vi "Getdata Loop.vi"(6 "Cluster Of Graphs":T1, 8 "error in":errorcluster, 9 "Reference For PLot":T2, 10 "User Event References":T3) -> (0 "error out":errorcluster)   [LabVIEW 2015]
uses:
  TypeDef/User Event References.ctl
  TypeDef/GetData Cluster.ctl
  TypeDef/ResultUpdate Cluster.ctl
  TypeDef/Initialize_Cluster.ctl
  TypeDef/OverWrite JSON Cluster.ctl
  TypeDef/UE Reference For Plot.ctl
  TypeDef/Plot Cluster.ctl
  TypeDef/GraphReff.ctl
  <vilib>/event_ctls.llb/usereventprio.ctl
  TypeDef/Shift Registers Cluster.ctl
  TypeDef/JSON Cluster(Int).ctl
  <vilib>/Utility/file.llb/Write Delimited Spreadsheet (string).vi
panel:
  out "Default Update Rate  3":enum16{"HIGH", "MEDIUM", "LOW"}(ring)
  out "Get Data Active 2":bool
  # "GetData Test Bench"
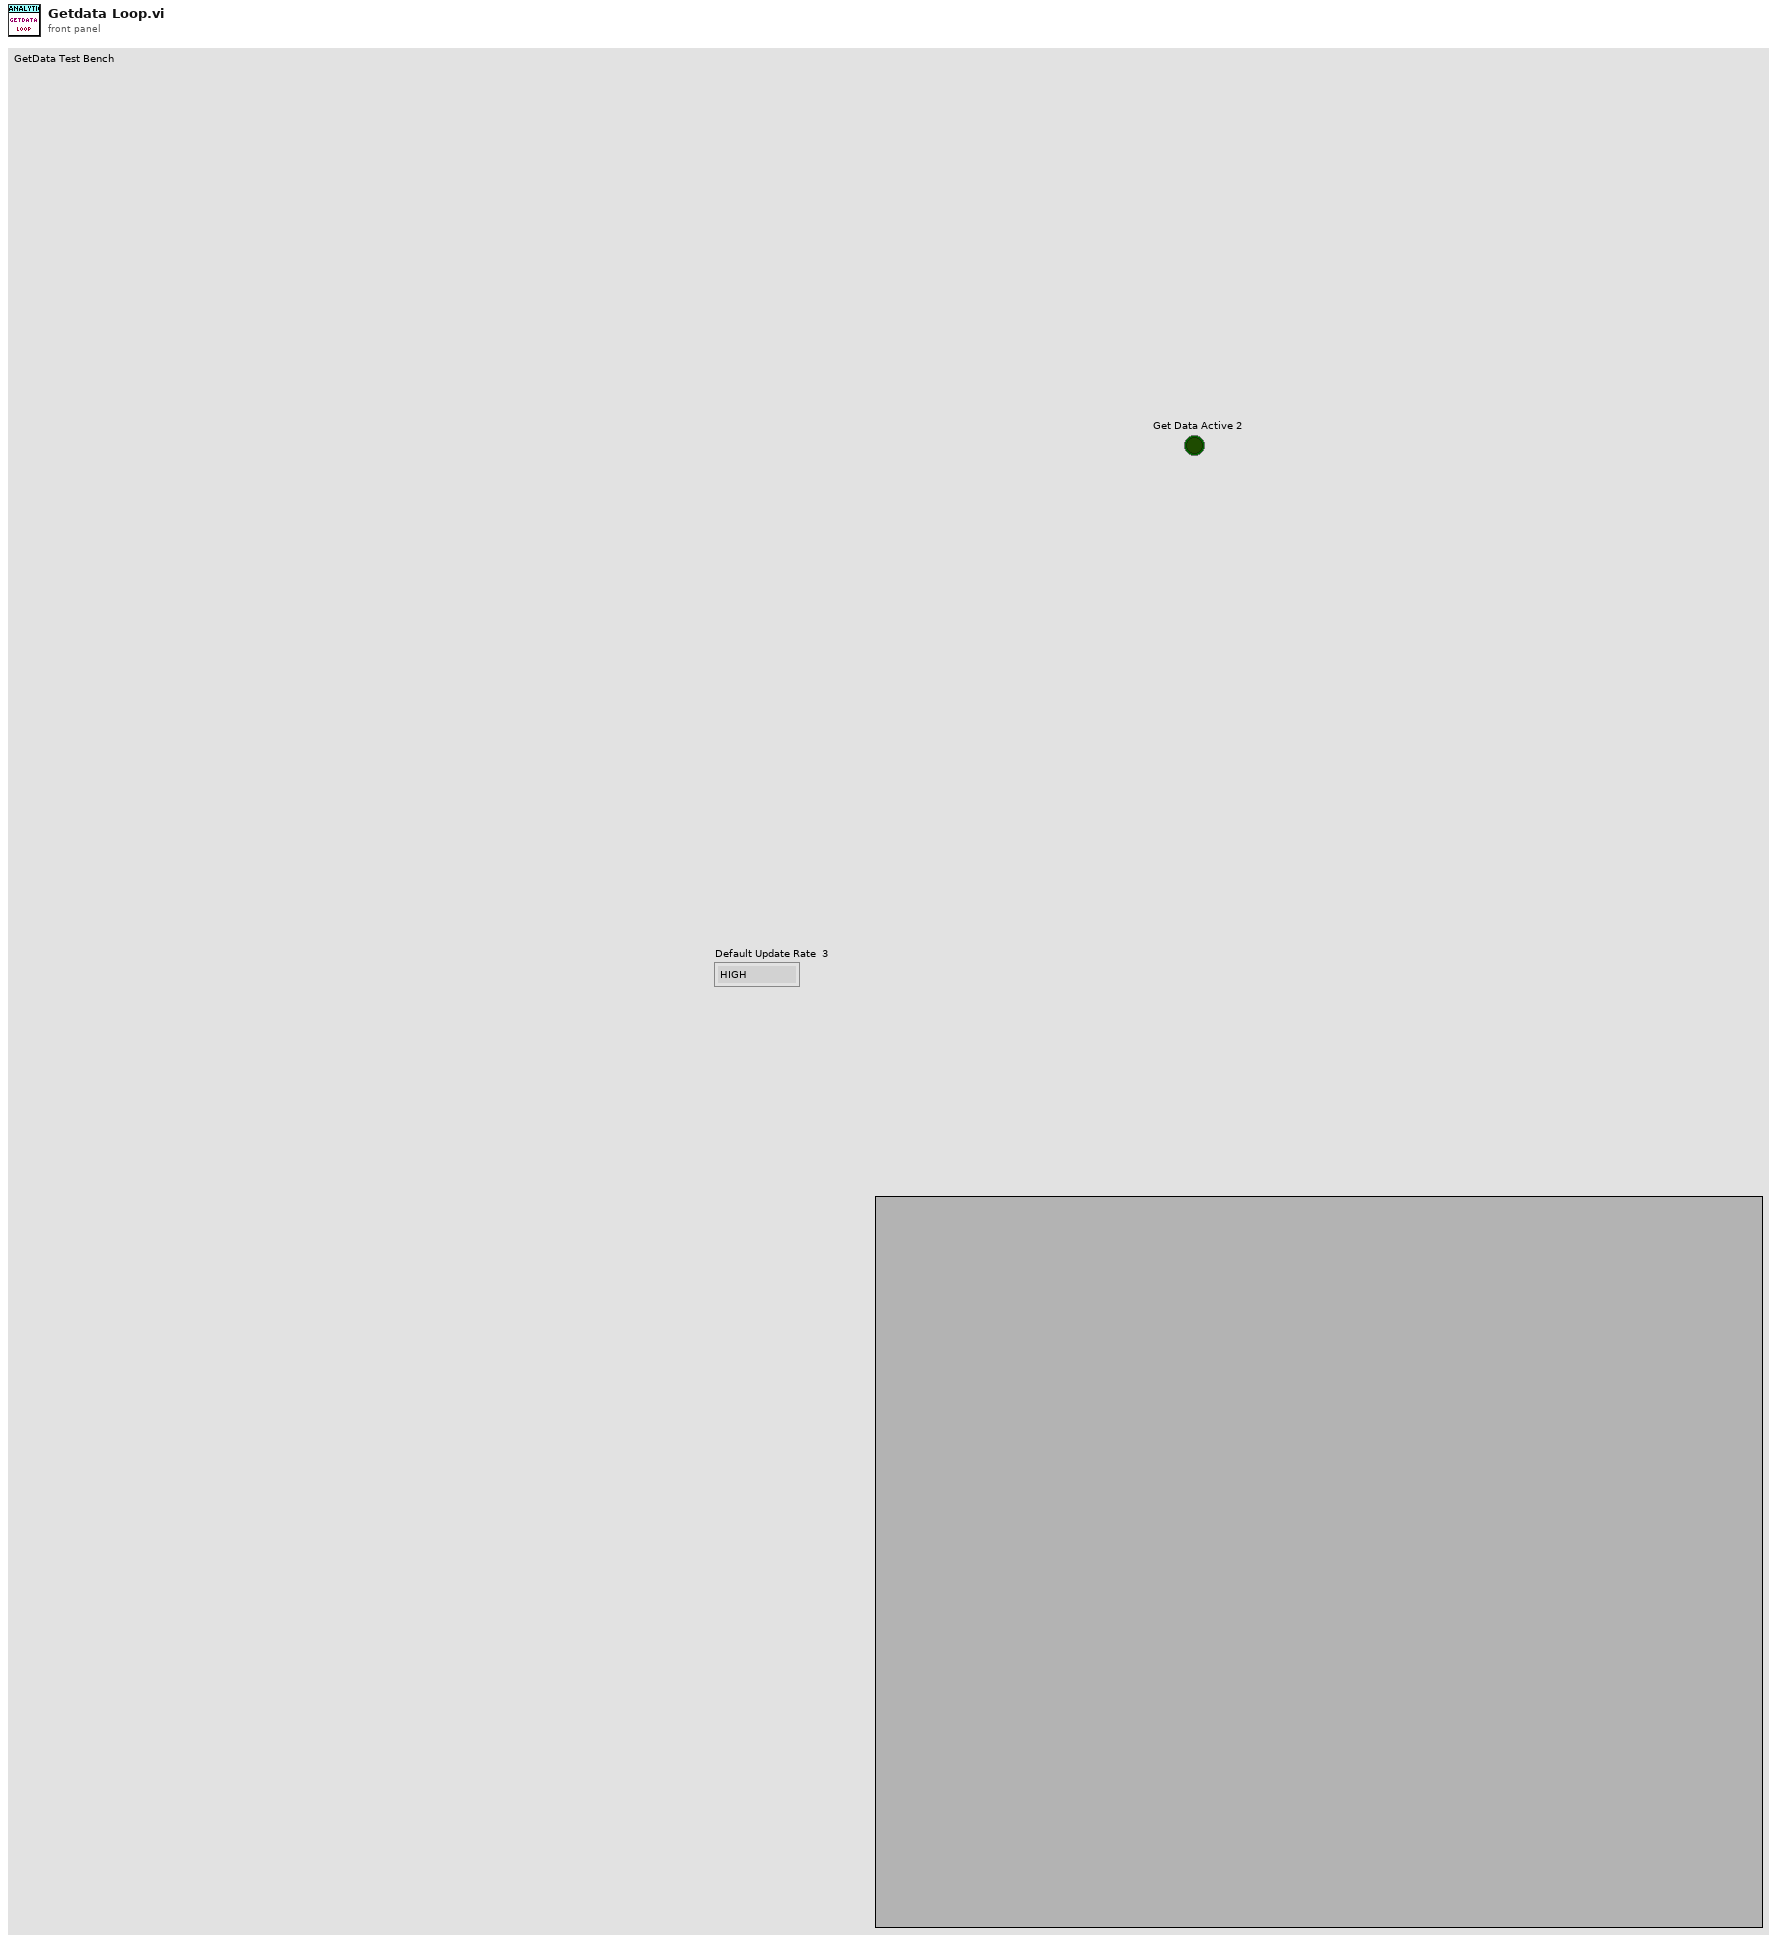
[diagram p1: front panel]
types:
  T1 = typedef "GraphReff.ctl" = cluster{"HistgramGraph-reff":refnum<vi>[], "BarGraph-reff":refnum<vi>[], "PieGraph-reff":refnum<vi>[], "Lable-reff":refnum<vi>[], "TrendGraph-reff":refnum<vi>[], "CpCpkTable":refnum<vi>}
  T2 = typedef "UE Reference For Plot.ctl" = cluster{"Stop_Plot":refnum<user-event>, "Exit_PLot":refnum<user-event>, "Plot":refnum<user-event>, "CpCpkData":refnum<user-event>}
  T3 = typedef "User Event References.ctl" = cluster{"Measurement":refnum<user-event>, "Stop_M":refnum<user-event>, "Exit_M":refnum<user-event>, "Analytics":refnum<user-event>, "Back":refnum<user-event>, "Getdata":refnum<user-event>, "ResultUpdate":refnum<user-event>, "Pause_M":refnum<user-event>, "Stop_Analytics":refnum<user-event>, "Exit_Analytics ":refnum<user-event>, "Measurement_M":refnum<user-event>, "Pause_Analytics":refnum<user-event>, "Initialization":refnum<user-event>, "Feedback_Pause":refnum<user-event>, "Feedback_Stop":refnum<user-event>, "Feedback_Exit":refnum<user-event>, "Override JSON":refnum<user-event>}
  T4 = typedef "usereventprio.ctl" = enum32{"high priority", "normal priority"}
  T5 = enum32{"invalid app kind", "Development System", "Run Time System", "Student Edition", "Embedded LabVIEW", "Evaluation", "Custom"}
  T6 = cluster{"AnalyticsParameters":cluster{"UpdateRateCategories":cluster{"LOW":cluster{"SampleElapsed":i32, "TimeElapsed":i32}, "MEDIUM":cluster{"SampleElapsed":i32, "TimeElapsed":i32}, "HIGH":cluster{"SampleElapsed":i32, "TimeElapsed":i32}}, "AnalyticsForPartsList":cluster{"Name":string, "InitializationValues":cluster{"RowsIn2DArray":i32, "ColumnsIn2DArray":i32, "SamplesToDisplay":i32, "UpdateRate":string}, "PlotParameters":cluster{"Trend":cluster{"TrendID":i32, "PlotEnable":bool, "PlotTitle":string, "PlotCaptionFont":cluster{"FontName":string, "FontSize":i32, "IsBold":bool, "IsItalic":bool, "IsUnderline":bool, "IsStrikeout":bool, "FontColor":string}, "XLabel":string, "XLabelFont":cluster{"FontName":string, "FontSize":i32, "IsBold":bool, "IsItalic":bool, "IsUnderline":bool, "IsStrikeout":bool, "FontColor":string}, "SamplesToDisplay":i32, "Channels":cluster{"Label":string, "YLabelFont":cluster{"FontName":string, "FontSize":i32, "IsBold":bool, "IsItalic":bool, "IsUnderline":bool, "IsStrikeout":bool, "FontColor":string}, "MeasurementID":i32, "PlotColor":string, "PointShape":string, "ShowOnGraph":bool}[]}[], "Histogram":cluster{"HistogramID":i32, "PlotEnable":bool, "PlotTitle":string, "PlotLabelFont":cluster{"FontName":string, "FontSize":i32, "IsBold":bool, "IsItalic":bool, "IsUnderline":bool, "IsStrikeout":bool, "FontColor":string}, "XLabel":string, "XLabelFont":cluster{"FontName":string, "FontSize":i32, "IsBold":bool, "IsItalic":bool, "IsUnderline":bool, "IsStrikeout":bool, "FontColor":string}, "YLabel":string, "YLabelFont":cluster{"FontName":string, "FontSize":i32, "IsBold":bool, "IsItalic":bool, "IsUnderline":bool, "IsStrikeout":bool, "FontColor":string}, "MeasurementID":i32, "PlotColor":string, "SamplesToDisplay":i32}[], "BarPlot":cluster{"BarPlotID":i32, "BarValuesID":i32, "PlotEnable":bool, "PlotLabel":string, "PlotLabelFont":cluster{"FontName":string, "FontSize":i32, "IsBold":bool, "IsItalic":bool, "IsUnderline":bool, "IsStrikeout":bool, "FontColor":string}, "XLabel":string, "XLabelFont":cluster{"FontName":string, "FontSize":i32, "IsBold":bool, "IsItalic":bool, "IsUnderline":bool, "IsStrikeout":bool, "FontColor":string}, "YLabel":string, "YLabelFont":cluster{"FontName":string, "FontSize":i32, "IsBold":bool, "IsItalic":bool, "IsUnderline":bool, "IsStrikeout":bool, "FontColor":string}, "Sectors":string[]}[], "PieChart":cluster{"PieChartID":i32, "PieChartValueID":i32, "PlotEnable":bool, "PlotLabel":string, "PlotLabelFont":cluster{"FontName":string, "FontSize":i32, "IsBold":bool, "IsItalic":bool, "IsUnderline":bool, "IsStrikeout":bool, "FontColor":string}, "Sectors":string[]}[]}}[]}}
  T7 = enum32{"Invalid", "Standard", "Closed", "Hidden", "Minimized", "Maximized"}
  T8 = cluster{"Terminal Count":u32, "isPass":bool, "Terminal Data 1D":dbl[], "Defect":bool[]}
  T9 = typedef "Shift Registers Cluster.ctl" = cluster{"Initialize 2D Array":dbl[][], "Analytics Button Pressed?":bool, "Analytics Or Back?":bool, "Read Config":bool, "Prev Terminal Count":u32, "Plot:Present Terminal":u32, "Timeout?":bool, "Re-initialized":bool}
  T10 = typedef "JSON Cluster(Int).ctl" = cluster{"Rows In 2D Array":i32, "Columns In 2D Array":i32, "Samples To Display":i32, "Update Rate (Time)":i32, "Update Rate (Samples)":i32, "MeasurementData":cluster{"MeasurementID":i32, "MeasureEnable":bool, "MeasurementPass":bool, "LimitSets":cluster{"LimitSetId":i32, "Limits":dbl[]}[]}[], "CurrentPartNumber":string, "AnalyticsDataFormat":cluster{"AnalyticsParameters":cluster{"UpdateRateCategories":cluster{"LOW":cluster{"SampleElapsed":i32, "TimeElapsed":i32}, "MEDIUM":cluster{"SampleElapsed":i32, "TimeElapsed":i32}, "HIGH":cluster{"SampleElapsed":i32, "TimeElapsed":i32}}, "AnalyticsForPartsList":cluster{"Name":string, "InitializationValues":cluster{"RowsIn2DArray":i32, "ColumnsIn2DArray":i32, "SamplesToDisplay":i32, "UpdateRate":string}, "PlotParameters":cluster{"Trend":cluster{"TrendID":i32, "PlotEnable":bool, "PlotTitle":string, "PlotCaptionFont":cluster{"FontName":string, "FontSize":i32, "IsBold":bool, "IsItalic":bool, "IsUnderline":bool, "IsStrikeout":bool, "FontColor":string}, "XLabel":string, "XLabelFont":cluster{"FontName":string, "FontSize":i32, "IsBold":bool, "IsItalic":bool, "IsUnderline":bool, "IsStrikeout":bool, "FontColor":string}, "SamplesToDisplay":i32, "Channels":cluster{"Label":string, "YLabelFont":cluster{"FontName":string, "FontSize":i32, "IsBold":bool, "IsItalic":bool, "IsUnderline":bool, "IsStrikeout":bool, "FontColor":string}, "MeasurementID":i32, "PlotColor":string, "PointShape":string, "ShowOnGraph":bool}[]}[], "Histogram":cluster{"HistogramID":i32, "PlotEnable":bool, "PlotTitle":string, "PlotLabelFont":cluster{"FontName":string, "FontSize":i32, "IsBold":bool, "IsItalic":bool, "IsUnderline":bool, "IsStrikeout":bool, "FontColor":string}, "XLabel":string, "XLabelFont":cluster{"FontName":string, "FontSize":i32, "IsBold":bool, "IsItalic":bool, "IsUnderline":bool, "IsStrikeout":bool, "FontColor":string}, "YLabel":string, "YLabelFont":cluster{"FontName":string, "FontSize":i32, "IsBold":bool, "IsItalic":bool, "IsUnderline":bool, "IsStrikeout":bool, "FontColor":string}, "MeasurementID":i32, "PlotColor":string, "SamplesToDisplay":i32}[], "BarPlot":cluster{"BarPlotID":i32, "BarValuesID":i32, "PlotEnable":bool, "PlotLabel":string, "PlotLabelFont":cluster{"FontName":string, "FontSize":i32, "IsBold":bool, "IsItalic":bool, "IsUnderline":bool, "IsStrikeout":bool, "FontColor":string}, "XLabel":string, "XLabelFont":cluster{"FontName":string, "FontSize":i32, "IsBold":bool, "IsItalic":bool, "IsUnderline":bool, "IsStrikeout":bool, "FontColor":string}, "YLabel":string, "YLabelFont":cluster{"FontName":string, "FontSize":i32, "IsBold":bool, "IsItalic":bool, "IsUnderline":bool, "IsStrikeout":bool, "FontColor":string}, "Sectors":string[]}[], "PieChart":cluster{"PieChartID":i32, "PieChartValueID":i32, "PlotEnable":bool, "PlotLabel":string, "PlotLabelFont":cluster{"FontName":string, "FontSize":i32, "IsBold":bool, "IsItalic":bool, "IsUnderline":bool, "IsStrikeout":bool, "FontColor":string}, "Sectors":string[]}[]}}[]}}, "PlotParameters":cluster{"Trend":cluster{"TrendID":i32, "PlotEnable":bool, "PlotTitle":string, "PlotCaptionFont":cluster{"FontName":string, "FontSize":i32, "IsBold":bool, "IsItalic":bool, "IsUnderline":bool, "IsStrikeout":bool, "FontColor":string}, "XLabel":string, "XLabelFont":cluster{"FontName":string, "FontSize":i32, "IsBold":bool, "IsItalic":bool, "IsUnderline":bool, "IsStrikeout":bool, "FontColor":string}, "SamplesToDisplay":i32, "Channels":cluster{"Label":string, "YLabelFont":cluster{"FontName":string, "FontSize":i32, "IsBold":bool, "IsItalic":bool, "IsUnderline":bool, "IsStrikeout":bool, "FontColor":string}, "MeasurementID":i32, "PlotColor":string, "PointShape":string, "ShowOnGraph":bool}[]}[], "Histogram":cluster{"HistogramID":i32, "PlotEnable":bool, "PlotTitle":string, "PlotLabelFont":cluster{"FontName":string, "FontSize":i32, "IsBold":bool, "IsItalic":bool, "IsUnderline":bool, "IsStrikeout":bool, "FontColor":string}, "XLabel":string, "XLabelFont":cluster{"FontName":string, "FontSize":i32, "IsBold":bool, "IsItalic":bool, "IsUnderline":bool, "IsStrikeout":bool, "FontColor":string}, "YLabel":string, "YLabelFont":cluster{"FontName":string, "FontSize":i32, "IsBold":bool, "IsItalic":bool, "IsUnderline":bool, "IsStrikeout":bool, "FontColor":string}, "MeasurementID":i32, "PlotColor":string, "SamplesToDisplay":i32}[], "BarPlot":cluster{"BarPlotID":i32, "BarValuesID":i32, "PlotEnable":bool, "PlotLabel":string, "PlotLabelFont":cluster{"FontName":string, "FontSize":i32, "IsBold":bool, "IsItalic":bool, "IsUnderline":bool, "IsStrikeout":bool, "FontColor":string}, "XLabel":string, "XLabelFont":cluster{"FontName":string, "FontSize":i32, "IsBold":bool, "IsItalic":bool, "IsUnderline":bool, "IsStrikeout":bool, "FontColor":string}, "YLabel":string, "YLabelFont":cluster{"FontName":string, "FontSize":i32, "IsBold":bool, "IsItalic":bool, "IsUnderline":bool, "IsStrikeout":bool, "FontColor":string}, "Sectors":string[]}[], "PieChart":cluster{"PieChartID":i32, "PieChartValueID":i32, "PlotEnable":bool, "PlotLabel":string, "PlotLabelFont":cluster{"FontName":string, "FontSize":i32, "IsBold":bool, "IsItalic":bool, "IsUnderline":bool, "IsStrikeout":bool, "FontColor":string}, "Sectors":string[]}[]}}
  T11 = cluster{"Core":cluster{"Current VI Reference":refnum<vi>, "Close Panel on Exit?":bool}, "clusterForShiftReg":T9, "JSON Cluster":T10, "AnalyticsDataFormat":cluster{"AnalyticsParameters":cluster{"UpdateRateCategories":cluster{"LOW":cluster{"SampleElapsed":i32, "TimeElapsed":i32}, "MEDIUM":cluster{"SampleElapsed":i32, "TimeElapsed":i32}, "HIGH":cluster{"SampleElapsed":i32, "TimeElapsed":i32}}, "AnalyticsForPartsList":cluster{"Name":string, "InitializationValues":cluster{"RowsIn2DArray":i32, "ColumnsIn2DArray":i32, "SamplesToDisplay":i32, "UpdateRate":string}, "PlotParameters":cluster{"Trend":cluster{"TrendID":i32, "PlotEnable":bool, "PlotTitle":string, "PlotCaptionFont":cluster{"FontName":string, "FontSize":i32, "IsBold":bool, "IsItalic":bool, "IsUnderline":bool, "IsStrikeout":bool, "FontColor":string}, "XLabel":string, "XLabelFont":cluster{"FontName":string, "FontSize":i32, "IsBold":bool, "IsItalic":bool, "IsUnderline":bool, "IsStrikeout":bool, "FontColor":string}, "SamplesToDisplay":i32, "Channels":cluster{"Label":string, "YLabelFont":cluster{"FontName":string, "FontSize":i32, "IsBold":bool, "IsItalic":bool, "IsUnderline":bool, "IsStrikeout":bool, "FontColor":string}, "MeasurementID":i32, "PlotColor":string, "PointShape":string, "ShowOnGraph":bool}[]}[], "Histogram":cluster{"HistogramID":i32, "PlotEnable":bool, "PlotTitle":string, "PlotLabelFont":cluster{"FontName":string, "FontSize":i32, "IsBold":bool, "IsItalic":bool, "IsUnderline":bool, "IsStrikeout":bool, "FontColor":string}, "XLabel":string, "XLabelFont":cluster{"FontName":string, "FontSize":i32, "IsBold":bool, "IsItalic":bool, "IsUnderline":bool, "IsStrikeout":bool, "FontColor":string}, "YLabel":string, "YLabelFont":cluster{"FontName":string, "FontSize":i32, "IsBold":bool, "IsItalic":bool, "IsUnderline":bool, "IsStrikeout":bool, "FontColor":string}, "MeasurementID":i32, "PlotColor":string, "SamplesToDisplay":i32}[], "BarPlot":cluster{"BarPlotID":i32, "BarValuesID":i32, "PlotEnable":bool, "PlotLabel":string, "PlotLabelFont":cluster{"FontName":string, "FontSize":i32, "IsBold":bool, "IsItalic":bool, "IsUnderline":bool, "IsStrikeout":bool, "FontColor":string}, "XLabel":string, "XLabelFont":cluster{"FontName":string, "FontSize":i32, "IsBold":bool, "IsItalic":bool, "IsUnderline":bool, "IsStrikeout":bool, "FontColor":string}, "YLabel":string, "YLabelFont":cluster{"FontName":string, "FontSize":i32, "IsBold":bool, "IsItalic":bool, "IsUnderline":bool, "IsStrikeout":bool, "FontColor":string}, "Sectors":string[]}[], "PieChart":cluster{"PieChartID":i32, "PieChartValueID":i32, "PlotEnable":bool, "PlotLabel":string, "PlotLabelFont":cluster{"FontName":string, "FontSize":i32, "IsBold":bool, "IsItalic":bool, "IsUnderline":bool, "IsStrikeout":bool, "FontColor":string}, "Sectors":string[]}[]}}[]}}, "Initialization Values":cluster{"InitializationParams":cluster{"CurrentPartNumber":string, "MeasurementData":cluster{"MeasurementID":i32, "MeasureEnable":bool, "MeasurementPass":bool, "LimitSets":cluster{"LimitSetId":i32, "Limits":dbl[]}[]}[]}}, "REsultCluster":cluster{"Terminal Count":u32, "isPass":bool, "Terminal Data 1D":dbl[], "Defect":bool[]}, "Pause Data":bool, "Statistical Parameters":string[][], "InitializationValues":dbl[][], "InitializationValue-PieCahrt":cluster{"InitializationDefect":dbl[], "InitializationProduction":dbl[]}, "InitializationValue-Barplot":cluster{"InitializationDefect":dbl[], "InitializationProduction":dbl[]}}
  T12 = cluster{"InitializationParams":cluster{"CurrentPartNumber":string, "MeasurementData":cluster{"MeasurementID":i32, "MeasureEnable":bool, "MeasurementPass":bool, "LimitSets":cluster{"LimitSetId":i32, "Limits":dbl[]}[]}[]}}
  T13 = typedef "Override JSON.ctl" = cluster{"AnalyticsDataFormat":cluster{"AnalyticsParameters":cluster{"UpdateRateCategories":cluster{"LOW":cluster{"SampleElapsed":i32, "TimeElapsed":i32}, "MEDIUM":cluster{"SampleElapsed":i32, "TimeElapsed":i32}, "HIGH":cluster{"SampleElapsed":i32, "TimeElapsed":i32}}, "AnalyticsForPartsList":cluster{"Name":string, "InitializationValues":cluster{"RowsIn2DArray":i32, "ColumnsIn2DArray":i32, "SamplesToDisplay":i32, "UpdateRate":string}, "PlotParameters":cluster{"Trend":cluster{"TrendID":i32, "PlotEnable":bool, "PlotTitle":string, "PlotCaptionFont":cluster{"FontName":string, "FontSize":i32, "IsBold":bool, "IsItalic":bool, "IsUnderline":bool, "IsStrikeout":bool, "FontColor":string}, "XLabel":string, "XLabelFont":cluster{"FontName":string, "FontSize":i32, "IsBold":bool, "IsItalic":bool, "IsUnderline":bool, "IsStrikeout":bool, "FontColor":string}, "SamplesToDisplay":i32, "Channels":cluster{"Label":string, "YLabelFont":cluster{"FontName":string, "FontSize":i32, "IsBold":bool, "IsItalic":bool, "IsUnderline":bool, "IsStrikeout":bool, "FontColor":string}, "MeasurementID":i32, "PlotColor":string, "PointShape":string, "ShowOnGraph":bool}[]}[], "Histogram":cluster{"HistogramID":i32, "PlotEnable":bool, "PlotTitle":string, "PlotLabelFont":cluster{"FontName":string, "FontSize":i32, "IsBold":bool, "IsItalic":bool, "IsUnderline":bool, "IsStrikeout":bool, "FontColor":string}, "XLabel":string, "XLabelFont":cluster{"FontName":string, "FontSize":i32, "IsBold":bool, "IsItalic":bool, "IsUnderline":bool, "IsStrikeout":bool, "FontColor":string}, "YLabel":string, "YLabelFont":cluster{"FontName":string, "FontSize":i32, "IsBold":bool, "IsItalic":bool, "IsUnderline":bool, "IsStrikeout":bool, "FontColor":string}, "MeasurementID":i32, "PlotColor":string, "SamplesToDisplay":i32}[], "BarPlot":cluster{"BarPlotID":i32, "BarValuesID":i32, "PlotEnable":bool, "PlotLabel":string, "PlotLabelFont":cluster{"FontName":string, "FontSize":i32, "IsBold":bool, "IsItalic":bool, "IsUnderline":bool, "IsStrikeout":bool, "FontColor":string}, "XLabel":string, "XLabelFont":cluster{"FontName":string, "FontSize":i32, "IsBold":bool, "IsItalic":bool, "IsUnderline":bool, "IsStrikeout":bool, "FontColor":string}, "YLabel":string, "YLabelFont":cluster{"FontName":string, "FontSize":i32, "IsBold":bool, "IsItalic":bool, "IsUnderline":bool, "IsStrikeout":bool, "FontColor":string}, "Sectors":string[]}[], "PieChart":cluster{"PieChartID":i32, "PieChartValueID":i32, "PlotEnable":bool, "PlotLabel":string, "PlotLabelFont":cluster{"FontName":string, "FontSize":i32, "IsBold":bool, "IsItalic":bool, "IsUnderline":bool, "IsStrikeout":bool, "FontColor":string}, "Sectors":string[]}[]}}[]}}}
  T14 = cluster{"InitializationDefect":dbl[], "InitializationProduction":dbl[]}
  T15 = cluster{"Current VI Reference":refnum<vi>, "Close Panel on Exit?":bool}
  T16 = cluster{"Trend":cluster{"TrendID":i32, "PlotEnable":bool, "PlotTitle":string, "PlotCaptionFont":cluster{"FontName":string, "FontSize":i32, "IsBold":bool, "IsItalic":bool, "IsUnderline":bool, "IsStrikeout":bool, "FontColor":string}, "XLabel":string, "XLabelFont":cluster{"FontName":string, "FontSize":i32, "IsBold":bool, "IsItalic":bool, "IsUnderline":bool, "IsStrikeout":bool, "FontColor":string}, "SamplesToDisplay":i32, "Channels":cluster{"Label":string, "YLabelFont":cluster{"FontName":string, "FontSize":i32, "IsBold":bool, "IsItalic":bool, "IsUnderline":bool, "IsStrikeout":bool, "FontColor":string}, "MeasurementID":i32, "PlotColor":string, "PointShape":string, "ShowOnGraph":bool}[]}[], "Histogram":cluster{"HistogramID":i32, "PlotEnable":bool, "PlotTitle":string, "PlotLabelFont":cluster{"FontName":string, "FontSize":i32, "IsBold":bool, "IsItalic":bool, "IsUnderline":bool, "IsStrikeout":bool, "FontColor":string}, "XLabel":string, "XLabelFont":cluster{"FontName":string, "FontSize":i32, "IsBold":bool, "IsItalic":bool, "IsUnderline":bool, "IsStrikeout":bool, "FontColor":string}, "YLabel":string, "YLabelFont":cluster{"FontName":string, "FontSize":i32, "IsBold":bool, "IsItalic":bool, "IsUnderline":bool, "IsStrikeout":bool, "FontColor":string}, "MeasurementID":i32, "PlotColor":string, "SamplesToDisplay":i32}[], "BarPlot":cluster{"BarPlotID":i32, "BarValuesID":i32, "PlotEnable":bool, "PlotLabel":string, "PlotLabelFont":cluster{"FontName":string, "FontSize":i32, "IsBold":bool, "IsItalic":bool, "IsUnderline":bool, "IsStrikeout":bool, "FontColor":string}, "XLabel":string, "XLabelFont":cluster{"FontName":string, "FontSize":i32, "IsBold":bool, "IsItalic":bool, "IsUnderline":bool, "IsStrikeout":bool, "FontColor":string}, "YLabel":string, "YLabelFont":cluster{"FontName":string, "FontSize":i32, "IsBold":bool, "IsItalic":bool, "IsUnderline":bool, "IsStrikeout":bool, "FontColor":string}, "Sectors":string[]}[], "PieChart":cluster{"PieChartID":i32, "PieChartValueID":i32, "PlotEnable":bool, "PlotLabel":string, "PlotLabelFont":cluster{"FontName":string, "FontSize":i32, "IsBold":bool, "IsItalic":bool, "IsUnderline":bool, "IsStrikeout":bool, "FontColor":string}, "Sectors":string[]}[]}
  T17 = cluster{"MeasurementID":i32, "MeasureEnable":bool, "MeasurementPass":bool, "LimitSets":cluster{"LimitSetId":i32, "Limits":dbl[]}[]}[]
  T18 = cluster{"Measurement-ID":i32[], "Measurement-Enable":bool[], "LSL":dbl[], "USL":dbl[]}
  T19 = typedef "Plot Cluster.ctl" = cluster{"Reduced 2D":dbl[][], "Start Index":i32, "MeasurementData":cluster{"MeasurementID":i32, "MeasureEnable":bool, "MeasurementPass":bool, "LimitSets":cluster{"LimitSetId":i32, "Limits":dbl[]}[]}[], "No Of New Termnals":i32, "Top/Bottom":bool, "Values Inserted":i32, "PlotParameters":cluster{"Trend":cluster{"TrendID":i32, "PlotEnable":bool, "PlotTitle":string, "PlotCaptionFont":cluster{"FontName":string, "FontSize":i32, "IsBold":bool, "IsItalic":bool, "IsUnderline":bool, "IsStrikeout":bool, "FontColor":string}, "XLabel":string, "XLabelFont":cluster{"FontName":string, "FontSize":i32, "IsBold":bool, "IsItalic":bool, "IsUnderline":bool, "IsStrikeout":bool, "FontColor":string}, "SamplesToDisplay":i32, "Channels":cluster{"Label":string, "YLabelFont":cluster{"FontName":string, "FontSize":i32, "IsBold":bool, "IsItalic":bool, "IsUnderline":bool, "IsStrikeout":bool, "FontColor":string}, "MeasurementID":i32, "PlotColor":string, "PointShape":string, "ShowOnGraph":bool}[]}[], "Histogram":cluster{"HistogramID":i32, "PlotEnable":bool, "PlotTitle":string, "PlotLabelFont":cluster{"FontName":string, "FontSize":i32, "IsBold":bool, "IsItalic":bool, "IsUnderline":bool, "IsStrikeout":bool, "FontColor":string}, "XLabel":string, "XLabelFont":cluster{"FontName":string, "FontSize":i32, "IsBold":bool, "IsItalic":bool, "IsUnderline":bool, "IsStrikeout":bool, "FontColor":string}, "YLabel":string, "YLabelFont":cluster{"FontName":string, "FontSize":i32, "IsBold":bool, "IsItalic":bool, "IsUnderline":bool, "IsStrikeout":bool, "FontColor":string}, "MeasurementID":i32, "PlotColor":string, "SamplesToDisplay":i32}[], "BarPlot":cluster{"BarPlotID":i32, "BarValuesID":i32, "PlotEnable":bool, "PlotLabel":string, "PlotLabelFont":cluster{"FontName":string, "FontSize":i32, "IsBold":bool, "IsItalic":bool, "IsUnderline":bool, "IsStrikeout":bool, "FontColor":string}, "XLabel":string, "XLabelFont":cluster{"FontName":string, "FontSize":i32, "IsBold":bool, "IsItalic":bool, "IsUnderline":bool, "IsStrikeout":bool, "FontColor":string}, "YLabel":string, "YLabelFont":cluster{"FontName":string, "FontSize":i32, "IsBold":bool, "IsItalic":bool, "IsUnderline":bool, "IsStrikeout":bool, "FontColor":string}, "Sectors":string[]}[], "PieChart":cluster{"PieChartID":i32, "PieChartValueID":i32, "PlotEnable":bool, "PlotLabel":string, "PlotLabelFont":cluster{"FontName":string, "FontSize":i32, "IsBold":bool, "IsItalic":bool, "IsUnderline":bool, "IsStrikeout":bool, "FontColor":string}, "Sectors":string[]}[]}, "Re-Initialised":bool, "Statistical params":string[][], "MeasurementData_IndexValues":cluster{"Measurement-ID":i32[], "Measurement-Enable":bool[], "LSL":dbl[], "USL":dbl[]}}
  T20 = cluster{"CurrentPartNumber":string, "MeasurementData":cluster{"MeasurementID":i32, "MeasureEnable":bool, "MeasurementPass":bool, "LimitSets":cluster{"LimitSetId":i32, "Limits":dbl[]}[]}[]}
  T21 = typedef "Json Partno Specific output.ctl" = cluster{"Array Params ":cluster{"RowsIn2DArray":i32, "ColumnsIn2DArray":i32, "SamplesToDisplay":i32, "UpdateRate":string}, "PlotParameters":cluster{"Trend":cluster{"TrendID":i32, "PlotEnable":bool, "PlotTitle":string, "PlotCaptionFont":cluster{"FontName":string, "FontSize":i32, "IsBold":bool, "IsItalic":bool, "IsUnderline":bool, "IsStrikeout":bool, "FontColor":string}, "XLabel":string, "XLabelFont":cluster{"FontName":string, "FontSize":i32, "IsBold":bool, "IsItalic":bool, "IsUnderline":bool, "IsStrikeout":bool, "FontColor":string}, "SamplesToDisplay":i32, "Channels":cluster{"Label":string, "YLabelFont":cluster{"FontName":string, "FontSize":i32, "IsBold":bool, "IsItalic":bool, "IsUnderline":bool, "IsStrikeout":bool, "FontColor":string}, "MeasurementID":i32, "PlotColor":string, "PointShape":string, "ShowOnGraph":bool}[]}[], "Histogram":cluster{"HistogramID":i32, "PlotEnable":bool, "PlotTitle":string, "PlotLabelFont":cluster{"FontName":string, "FontSize":i32, "IsBold":bool, "IsItalic":bool, "IsUnderline":bool, "IsStrikeout":bool, "FontColor":string}, "XLabel":string, "XLabelFont":cluster{"FontName":string, "FontSize":i32, "IsBold":bool, "IsItalic":bool, "IsUnderline":bool, "IsStrikeout":bool, "FontColor":string}, "YLabel":string, "YLabelFont":cluster{"FontName":string, "FontSize":i32, "IsBold":bool, "IsItalic":bool, "IsUnderline":bool, "IsStrikeout":bool, "FontColor":string}, "MeasurementID":i32, "PlotColor":string, "SamplesToDisplay":i32}[], "BarPlot":cluster{"BarPlotID":i32, "BarValuesID":i32, "PlotEnable":bool, "PlotLabel":string, "PlotLabelFont":cluster{"FontName":string, "FontSize":i32, "IsBold":bool, "IsItalic":bool, "IsUnderline":bool, "IsStrikeout":bool, "FontColor":string}, "XLabel":string, "XLabelFont":cluster{"FontName":string, "FontSize":i32, "IsBold":bool, "IsItalic":bool, "IsUnderline":bool, "IsStrikeout":bool, "FontColor":string}, "YLabel":string, "YLabelFont":cluster{"FontName":string, "FontSize":i32, "IsBold":bool, "IsItalic":bool, "IsUnderline":bool, "IsStrikeout":bool, "FontColor":string}, "Sectors":string[]}[], "PieChart":cluster{"PieChartID":i32, "PieChartValueID":i32, "PlotEnable":bool, "PlotLabel":string, "PlotLabelFont":cluster{"FontName":string, "FontSize":i32, "IsBold":bool, "IsItalic":bool, "IsUnderline":bool, "IsStrikeout":bool, "FontColor":string}, "Sectors":string[]}[]}}
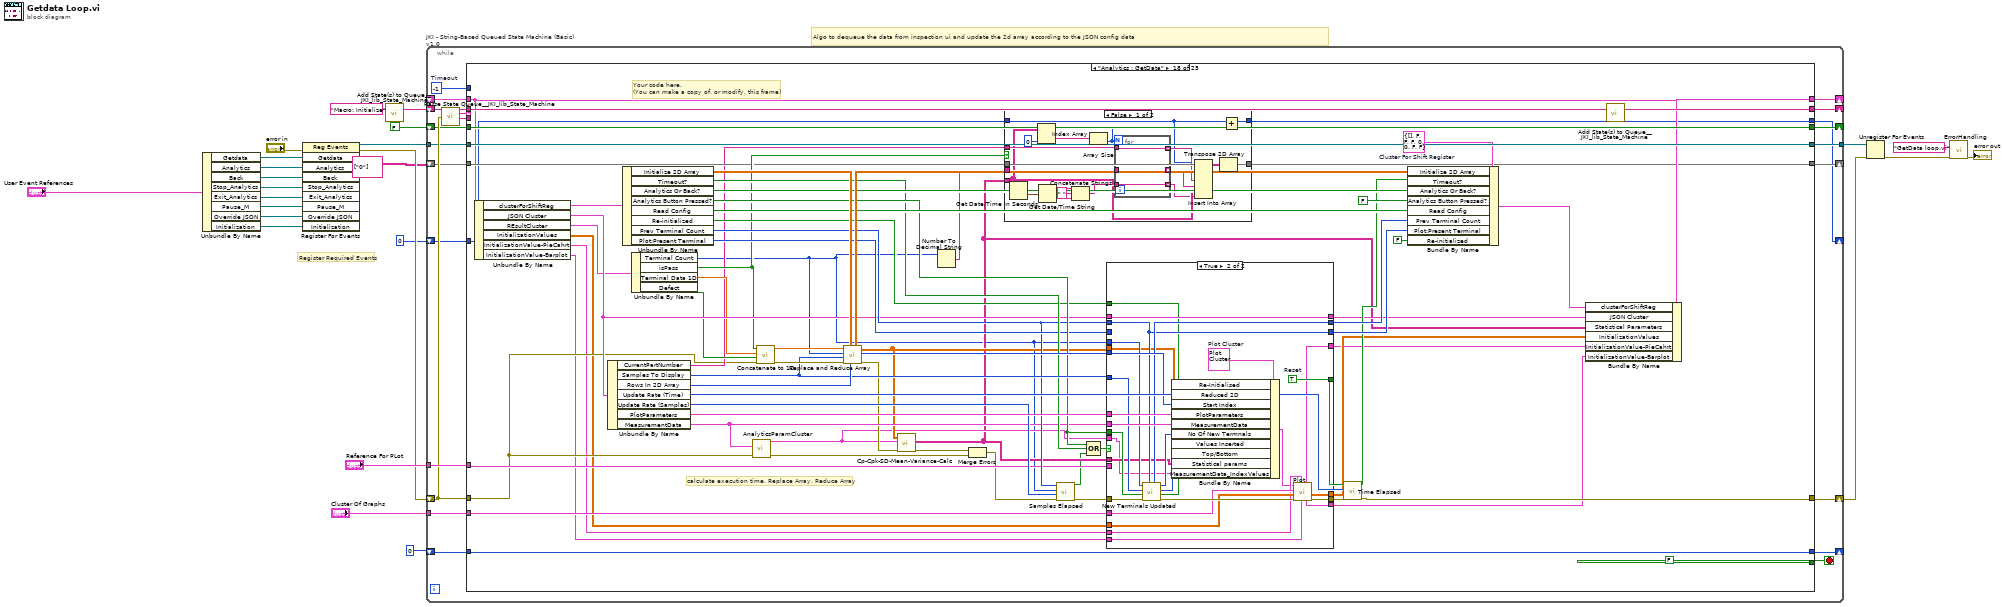
[diagram p0: block diagram]
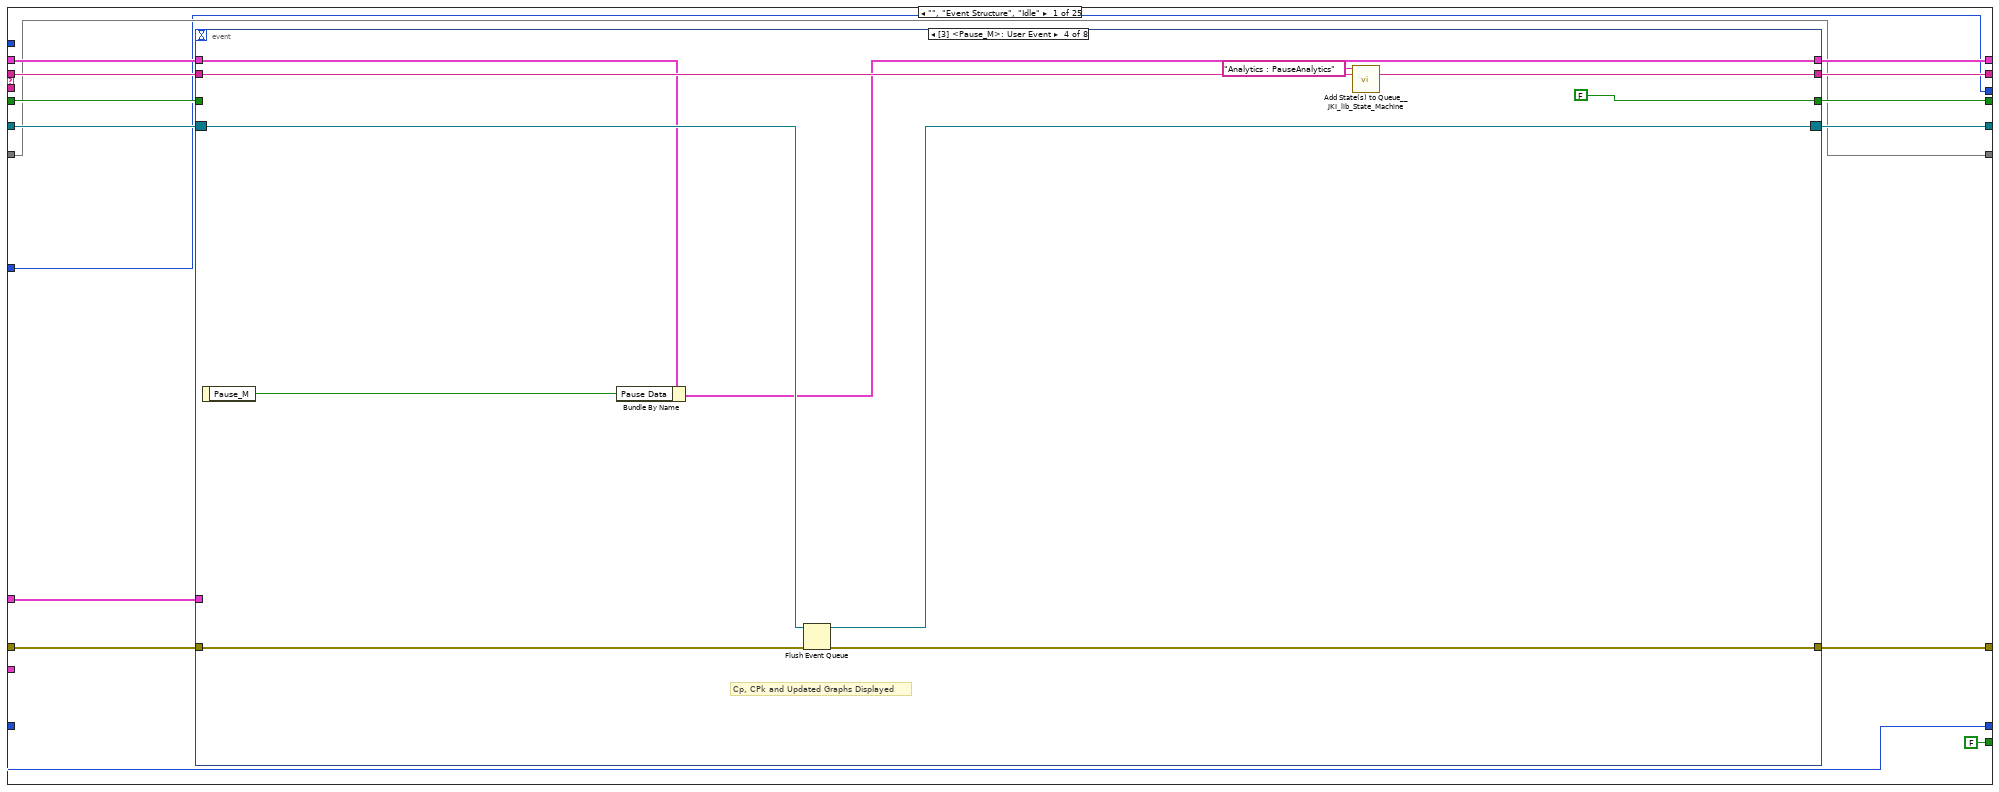
[diagram p2: hidden frame]
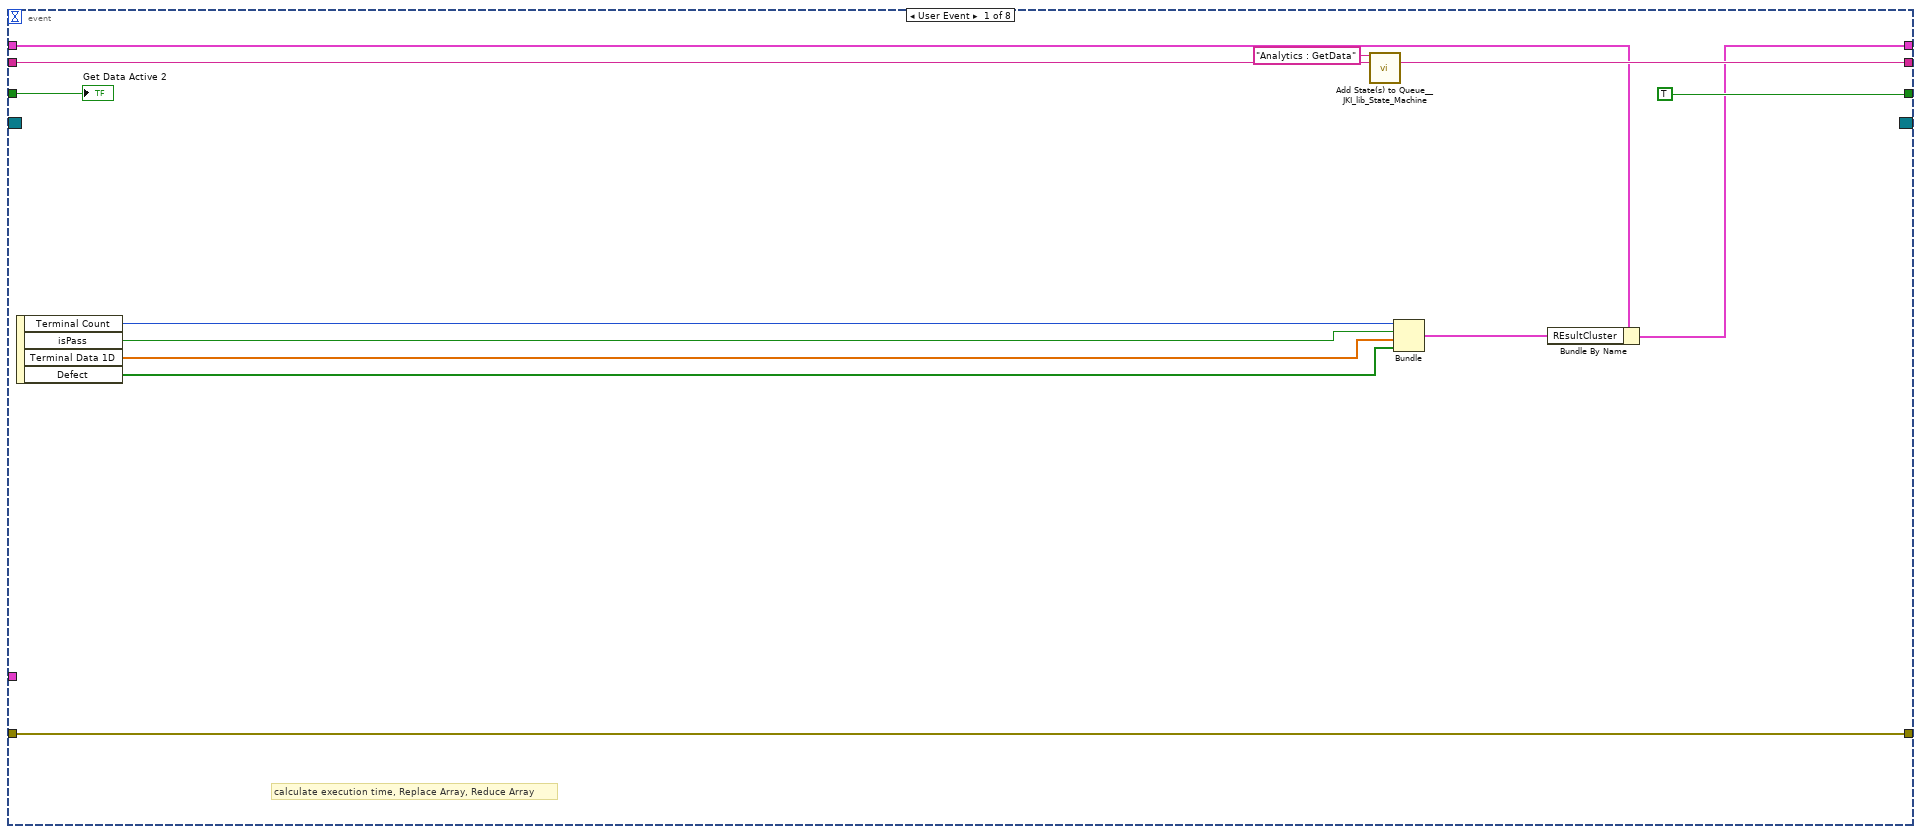
[diagram p3: hidden frame]
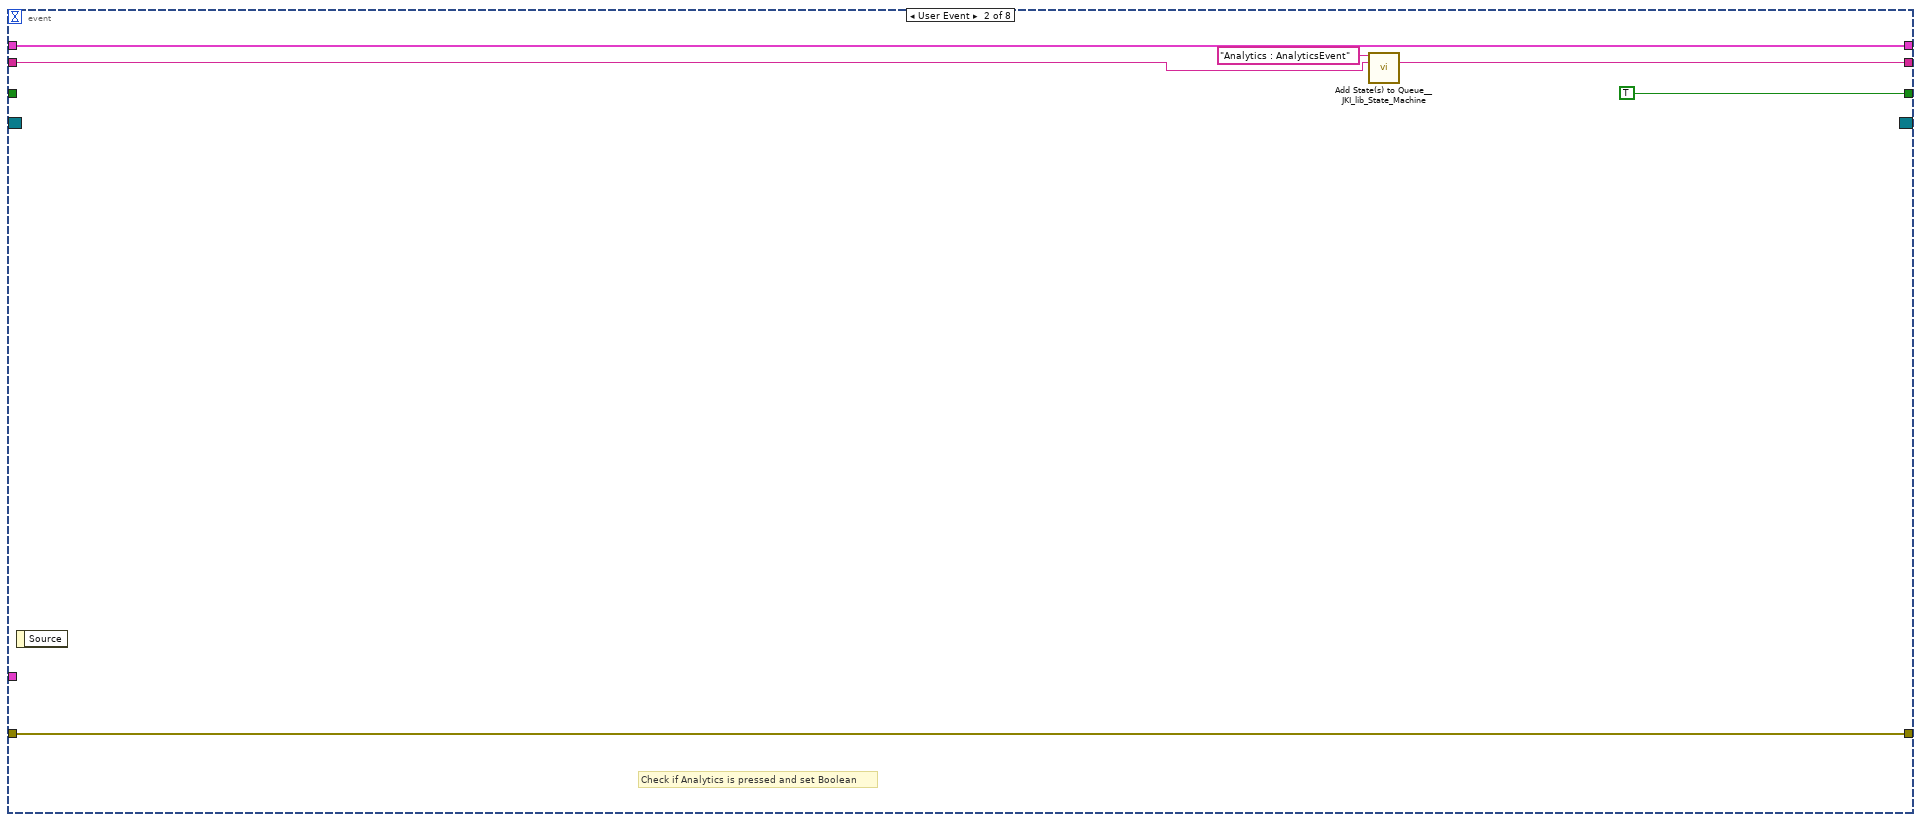
[diagram p4: hidden frame]
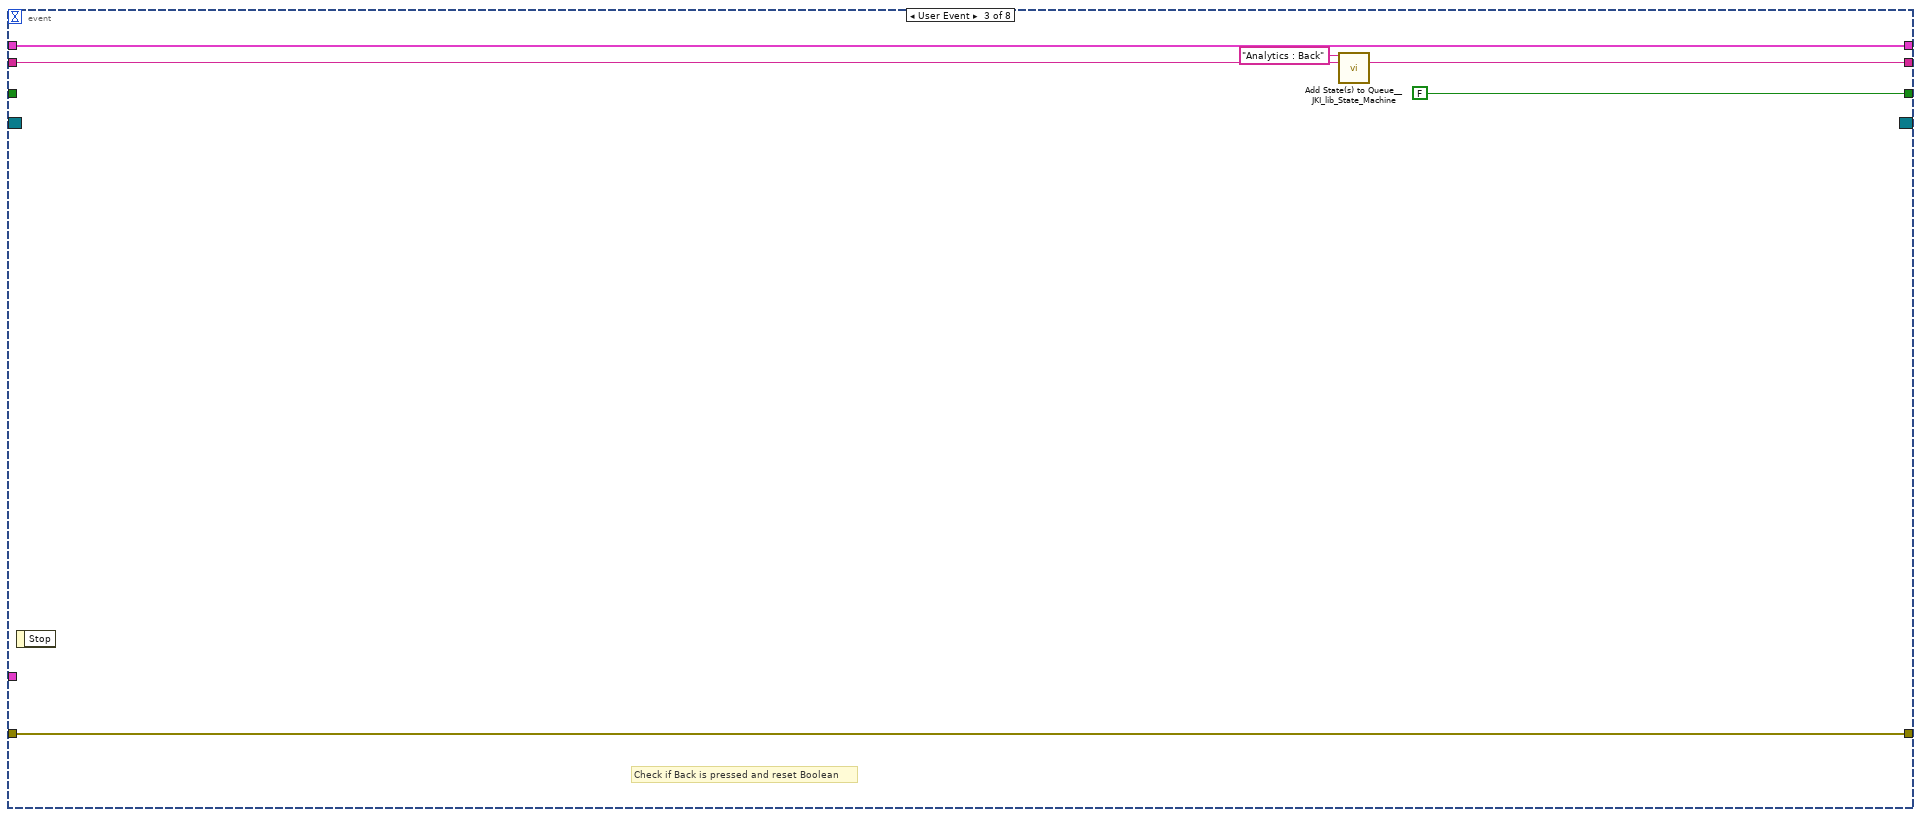
[diagram p5: hidden frame]
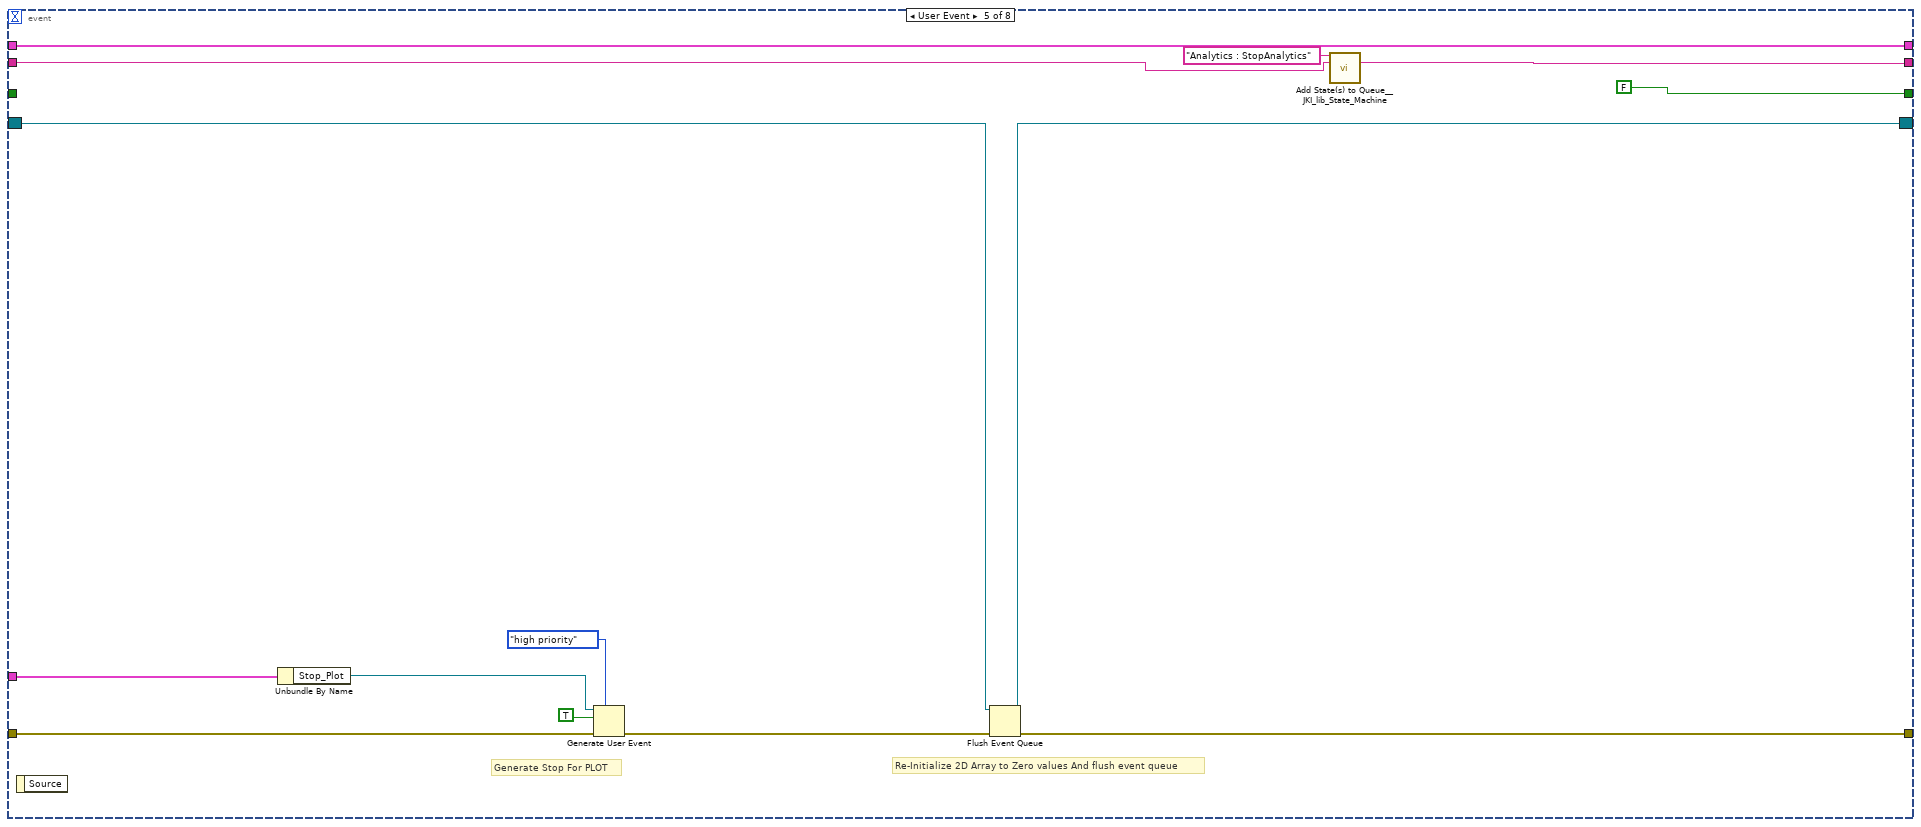
[diagram p6: hidden frame]
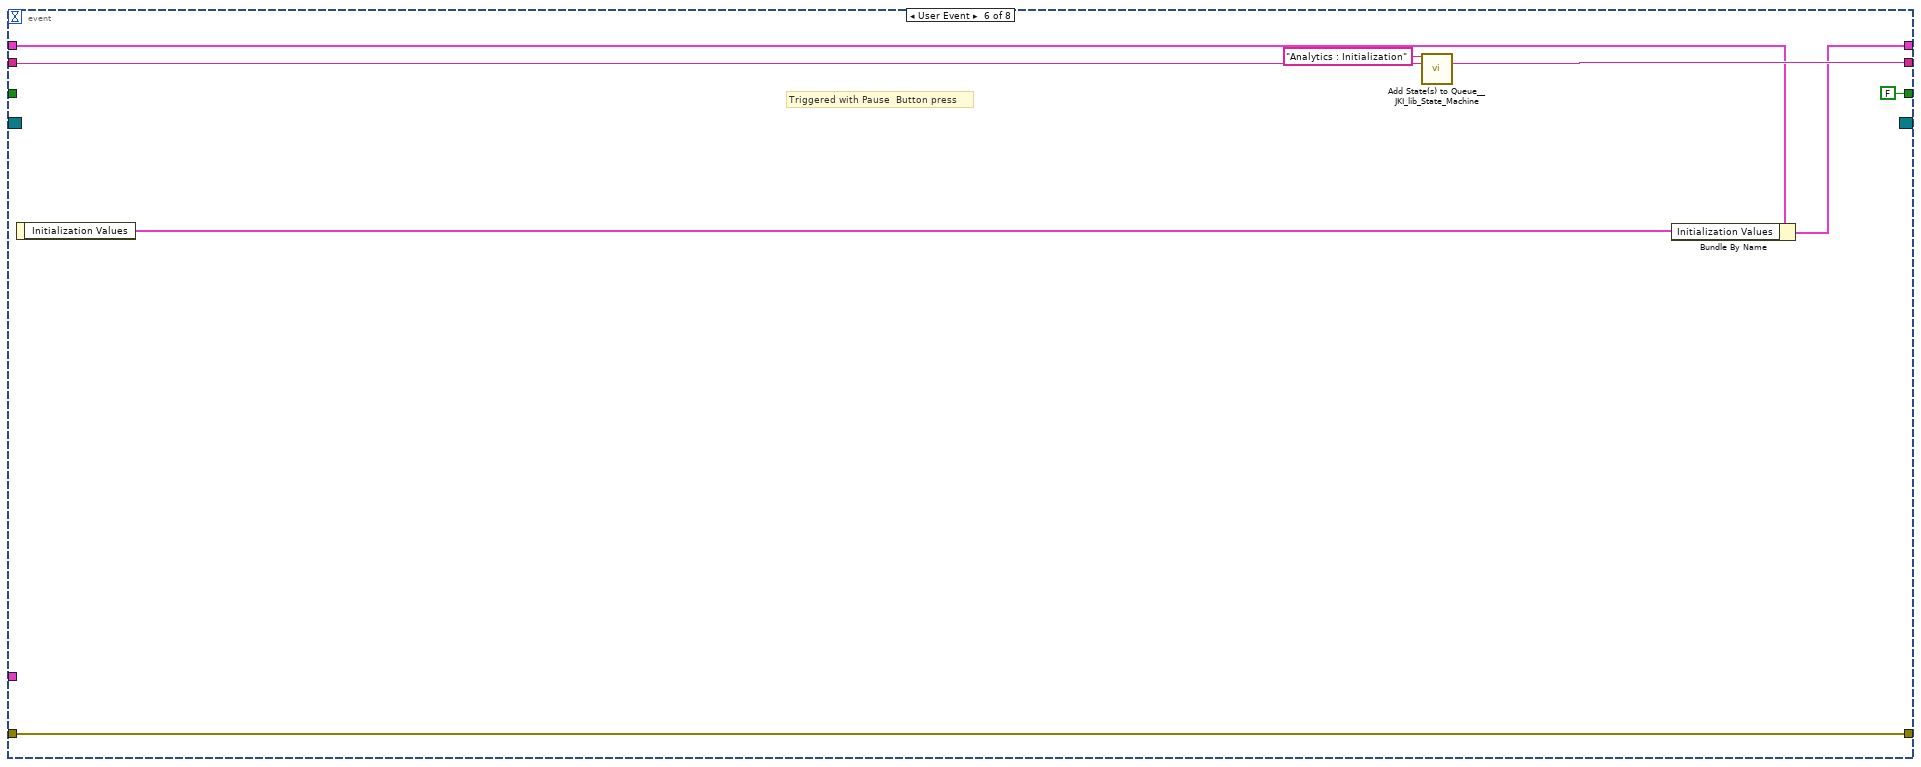
[diagram p7: hidden frame]
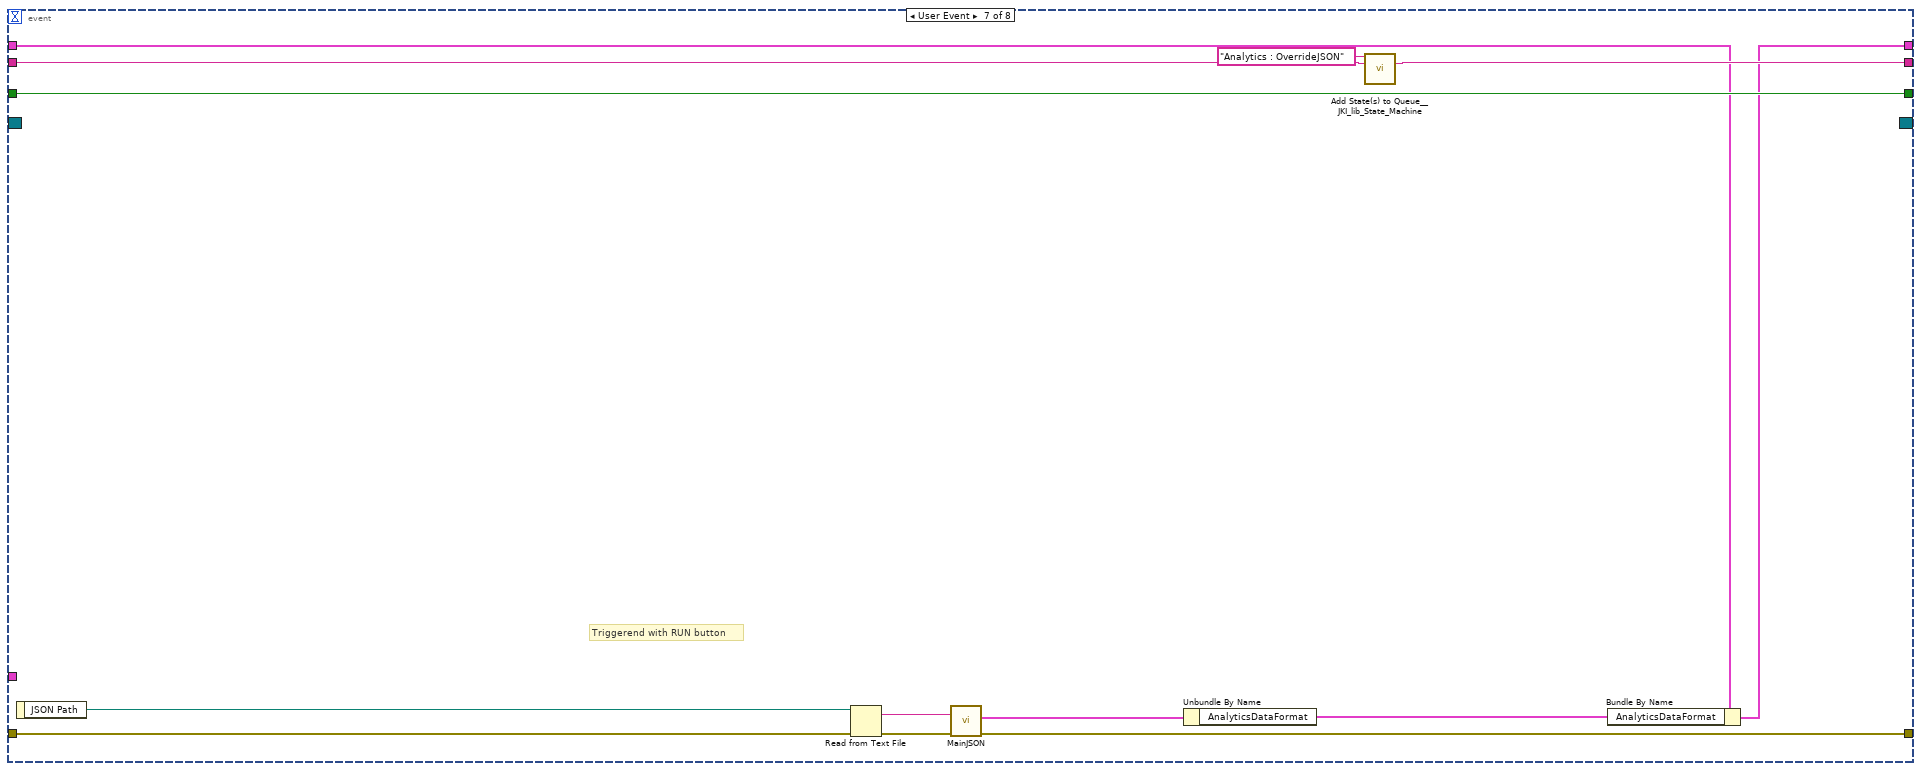
[diagram p8: hidden frame]
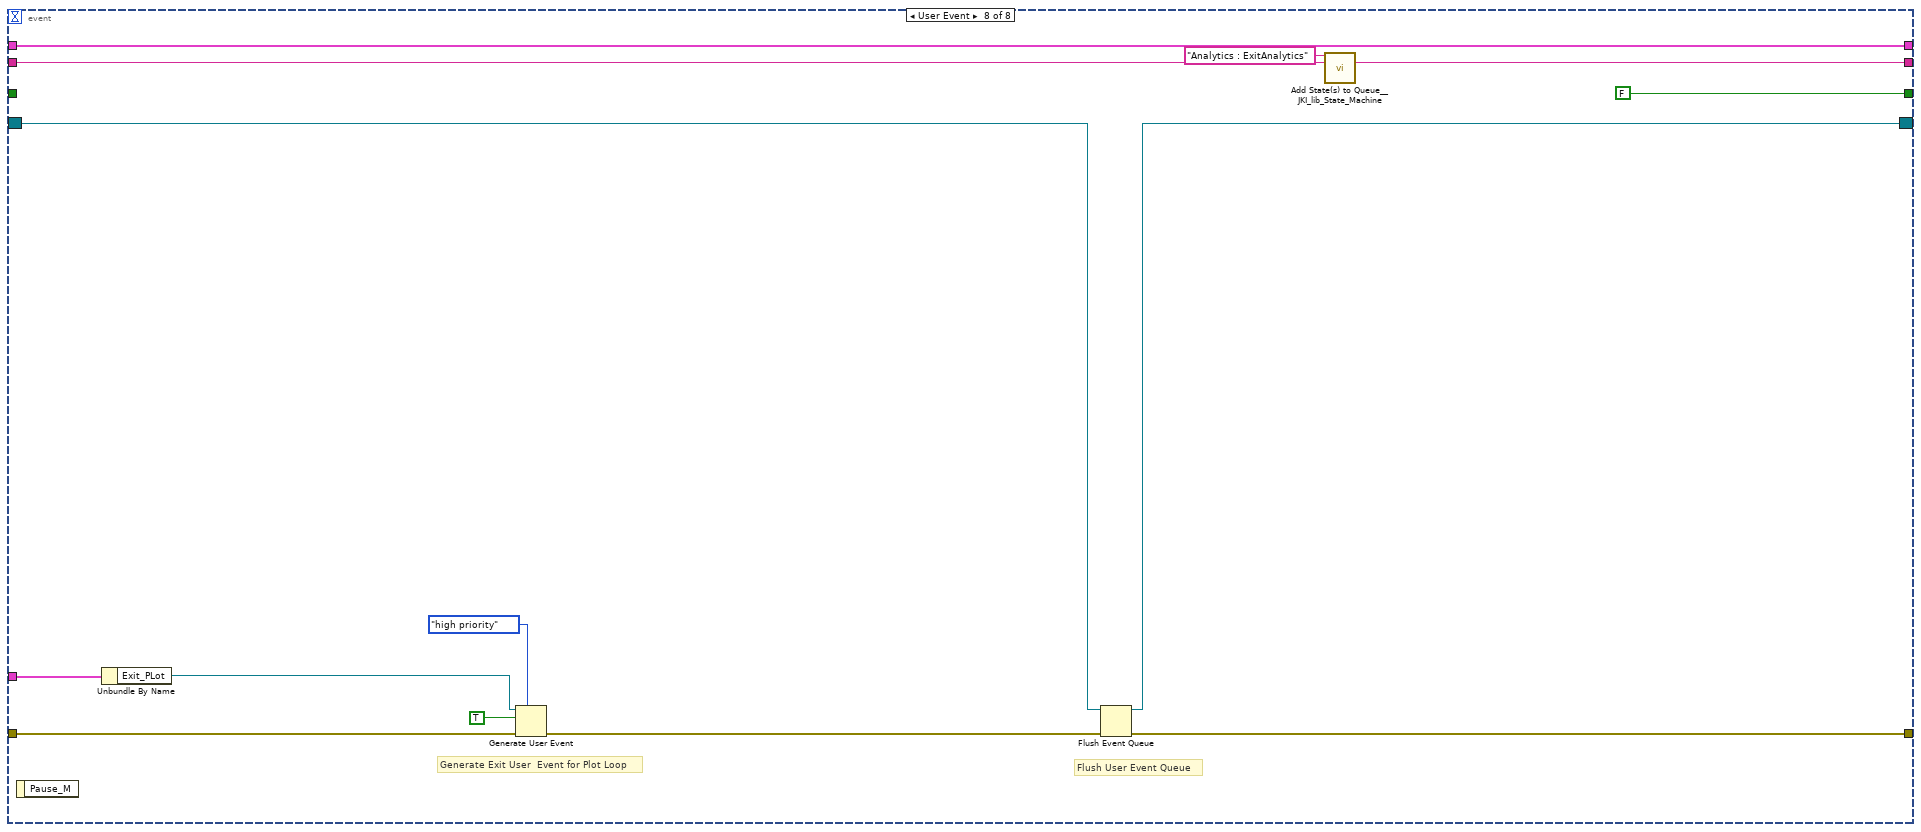
[diagram p9: hidden frame]
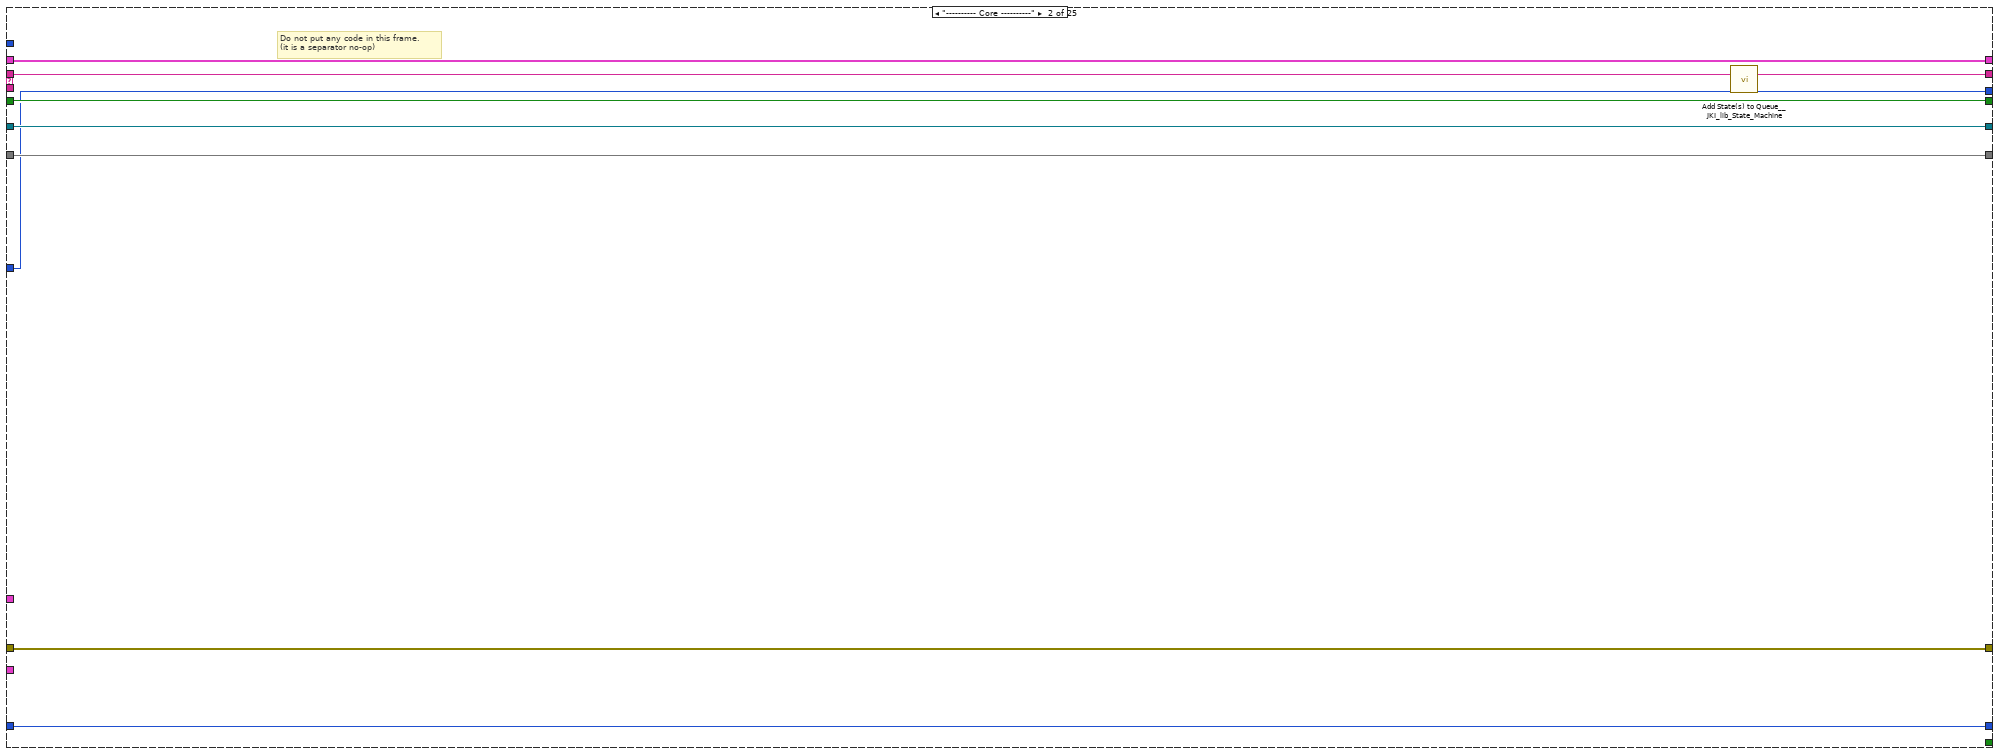
[diagram p10: hidden frame]
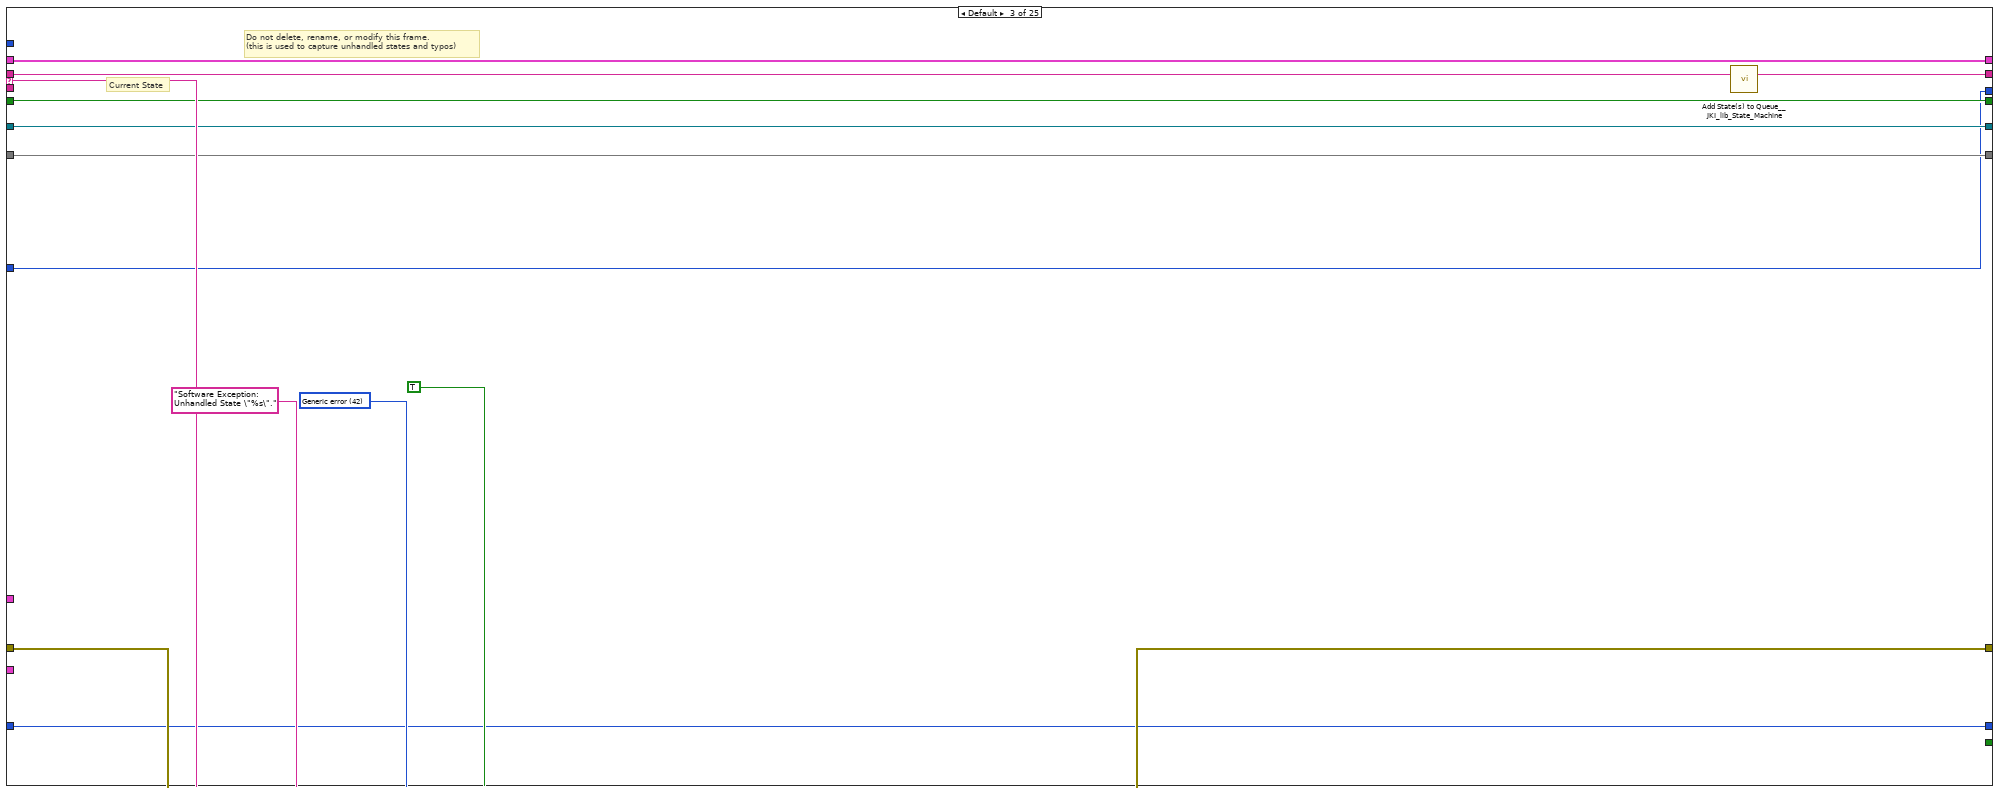
[diagram p11: hidden frame]
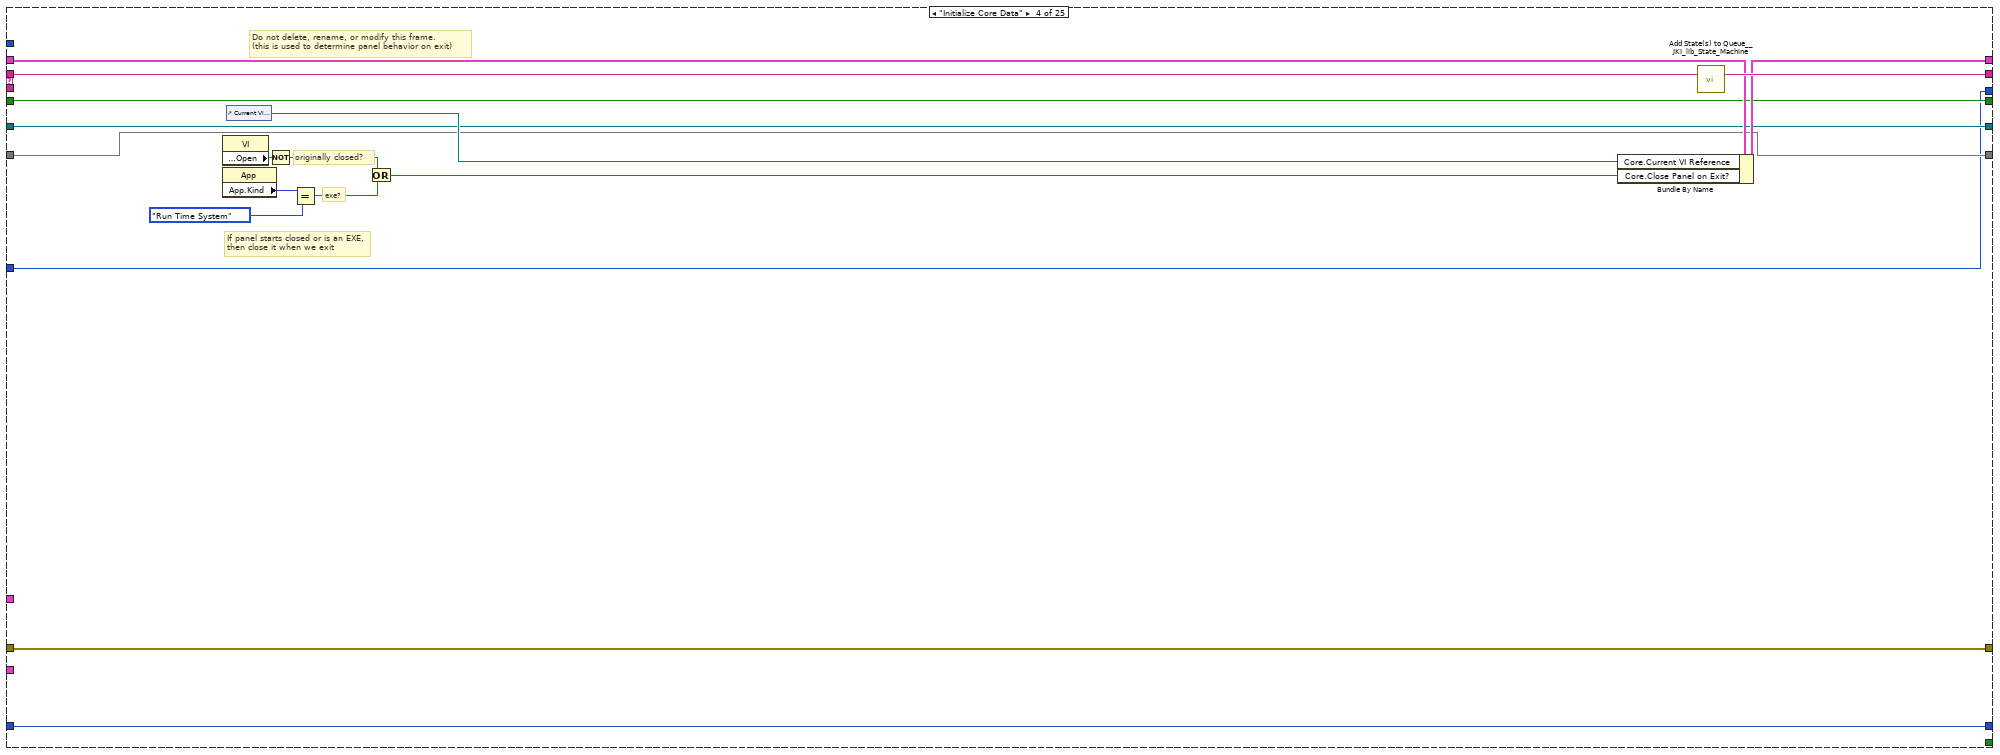
[diagram p12: hidden frame]
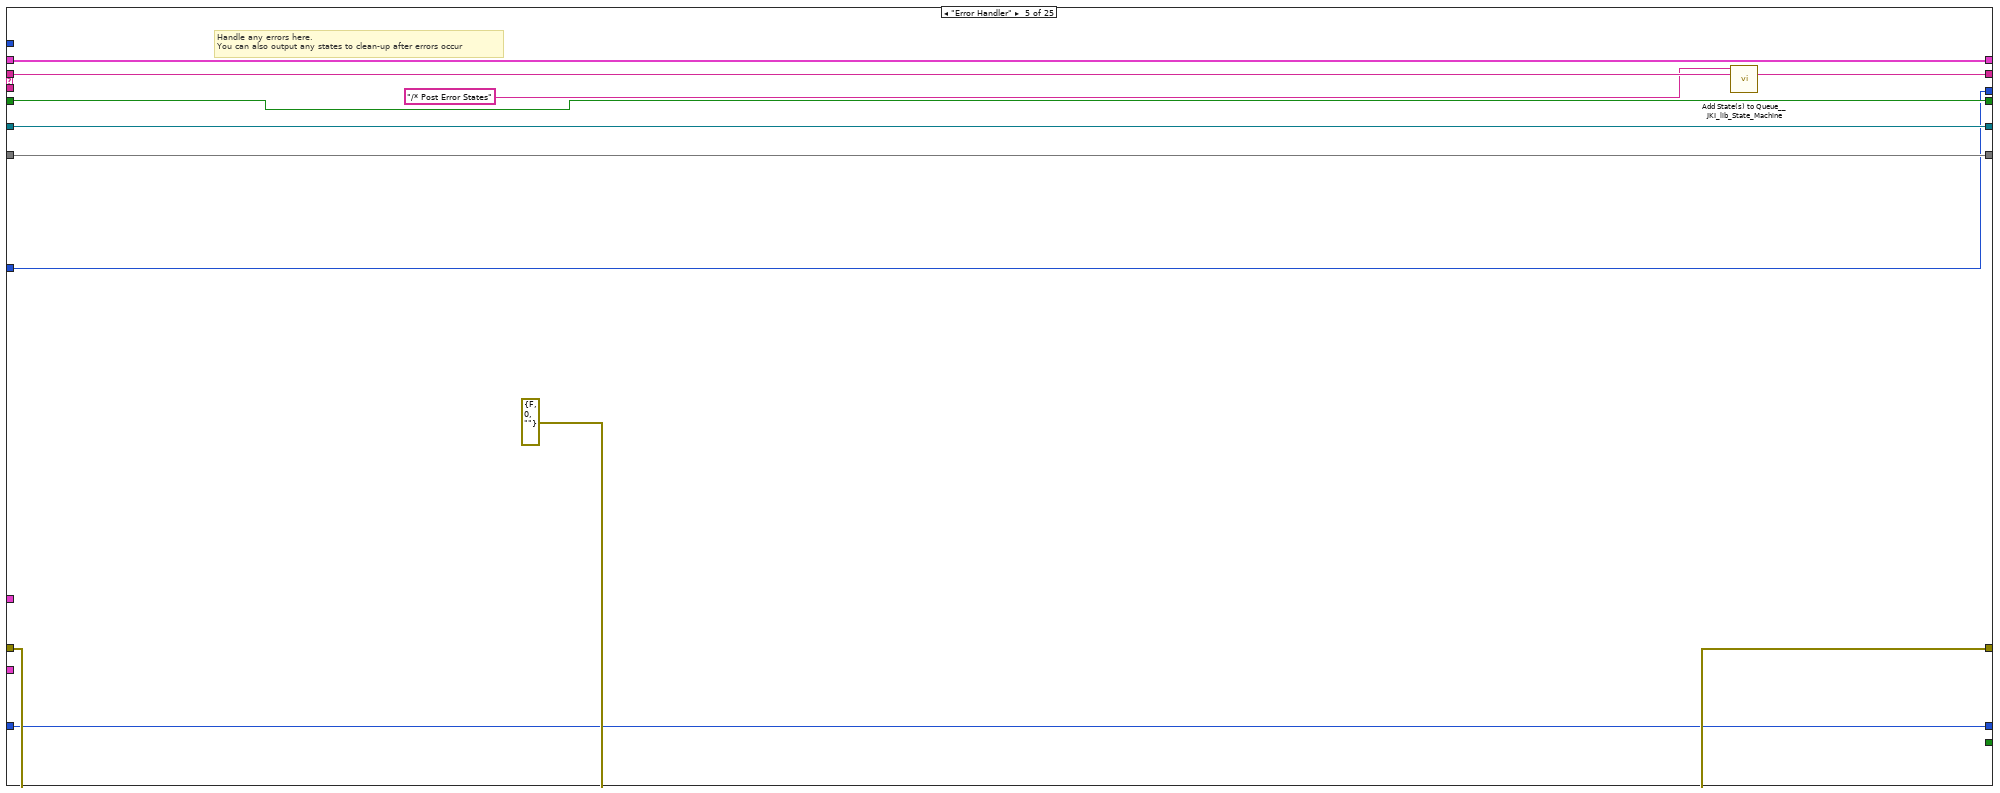
[diagram p13: hidden frame]
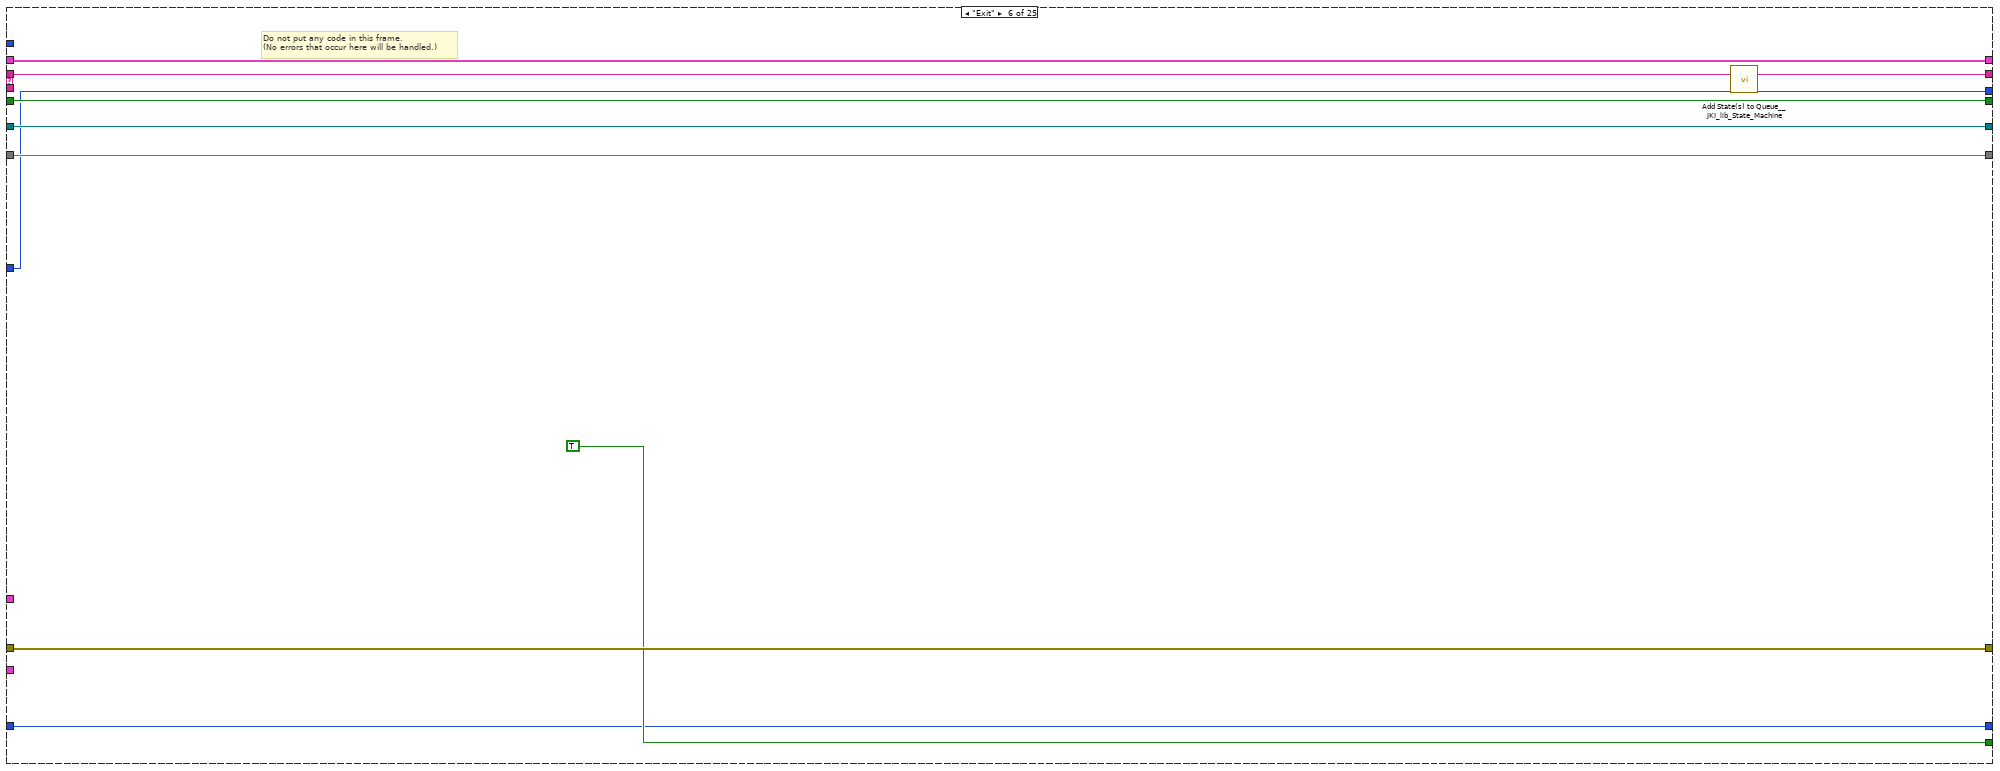
[diagram p14: hidden frame]
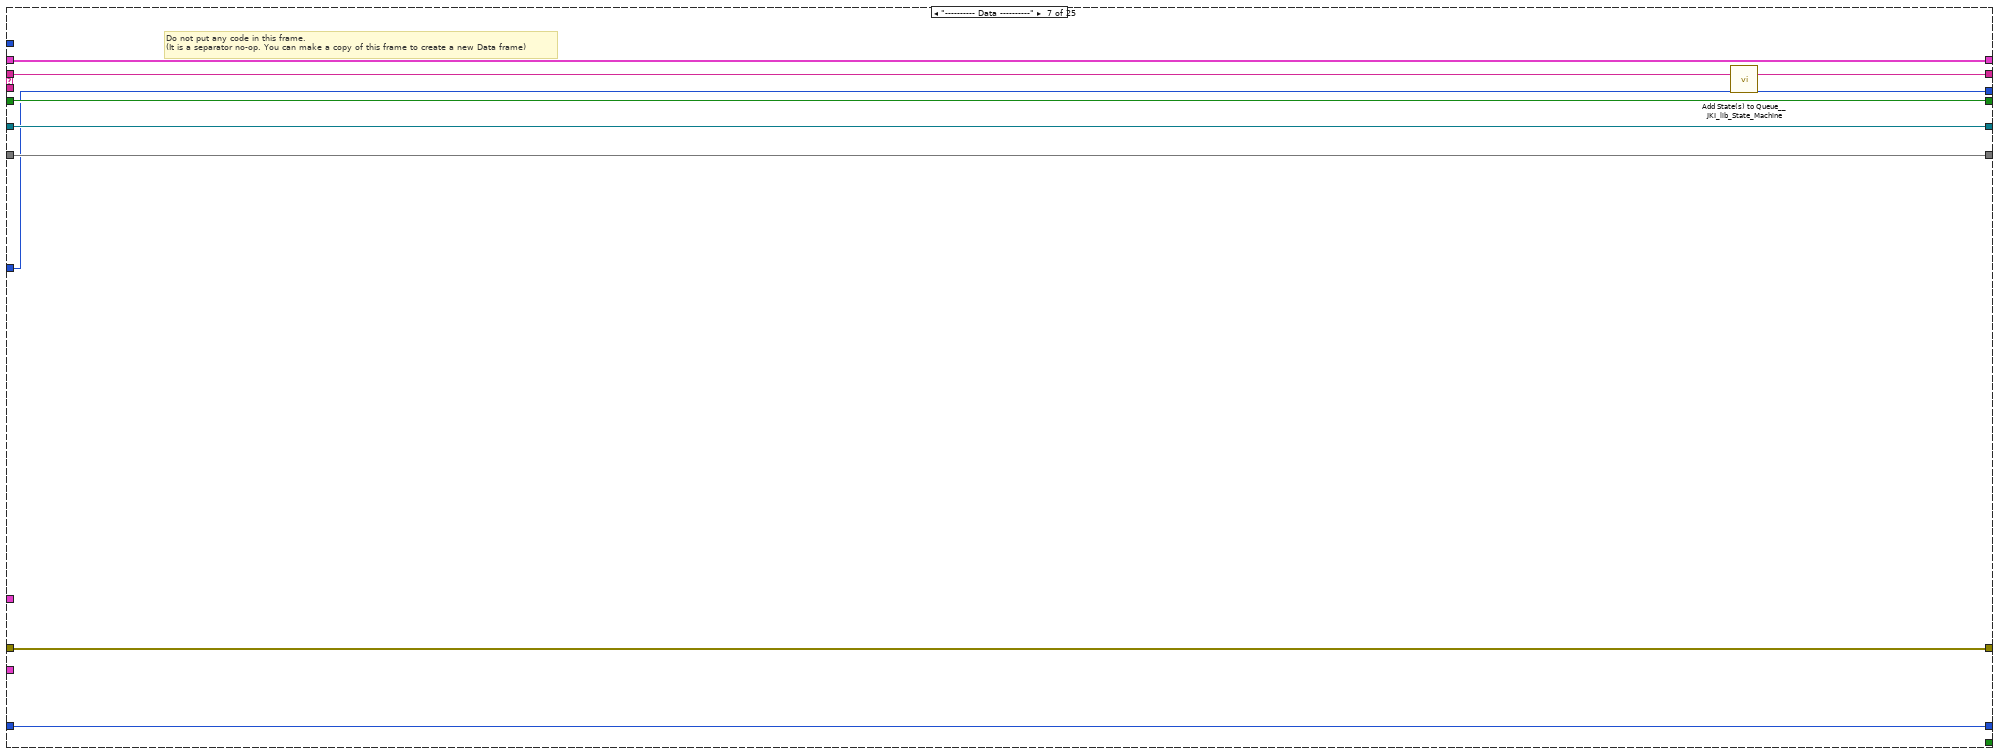
[diagram p15: hidden frame]
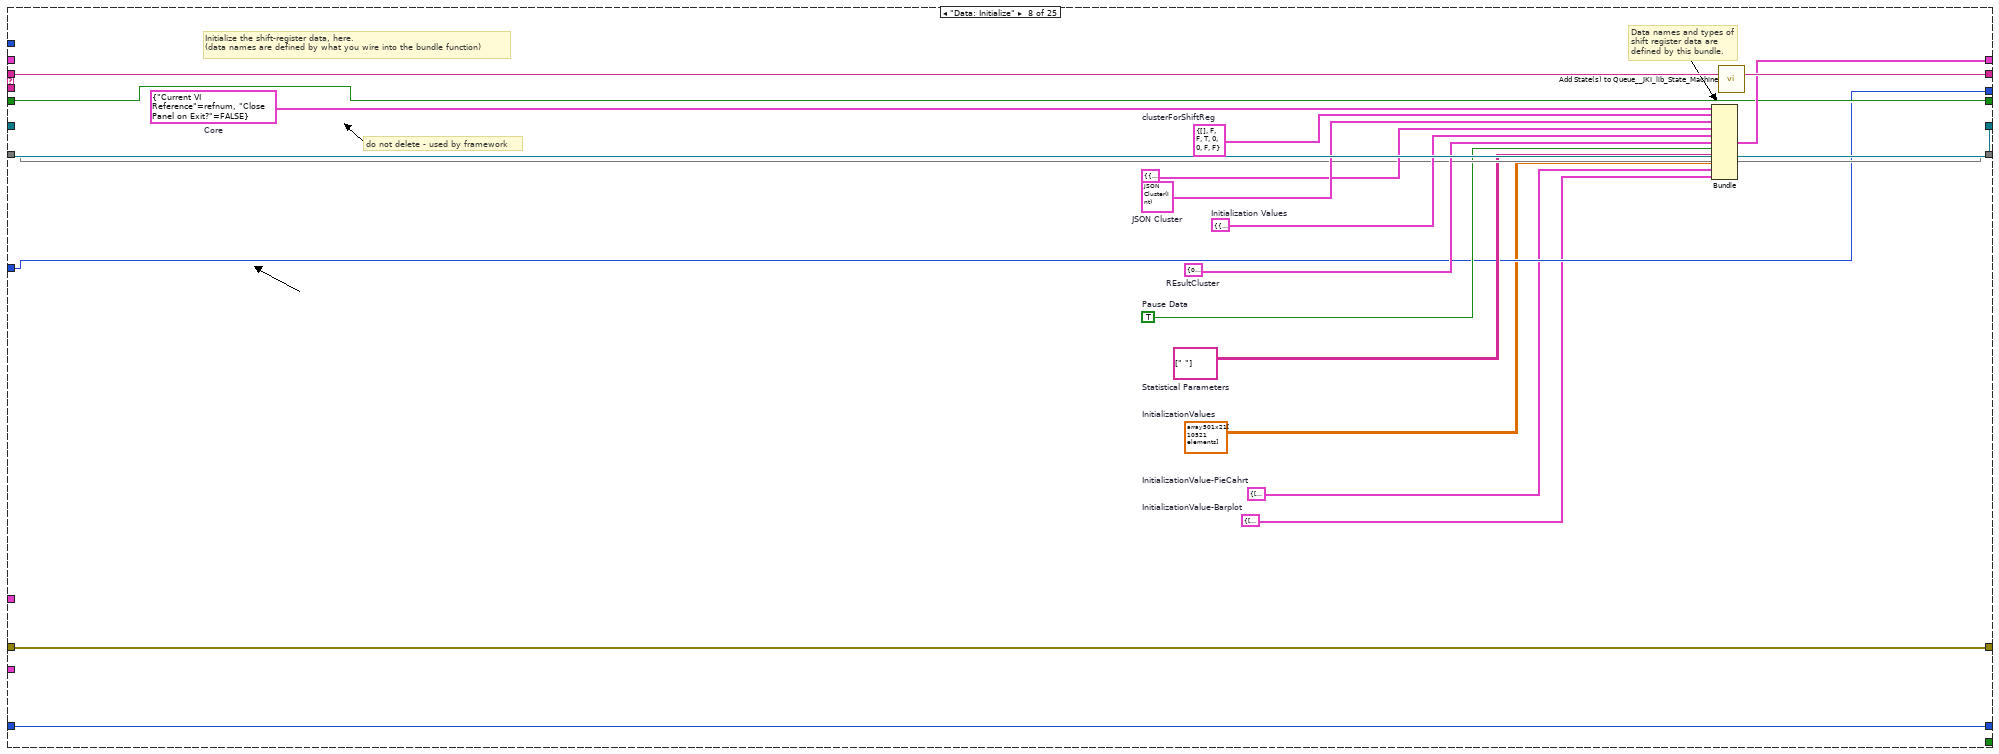
[diagram p16: hidden frame]
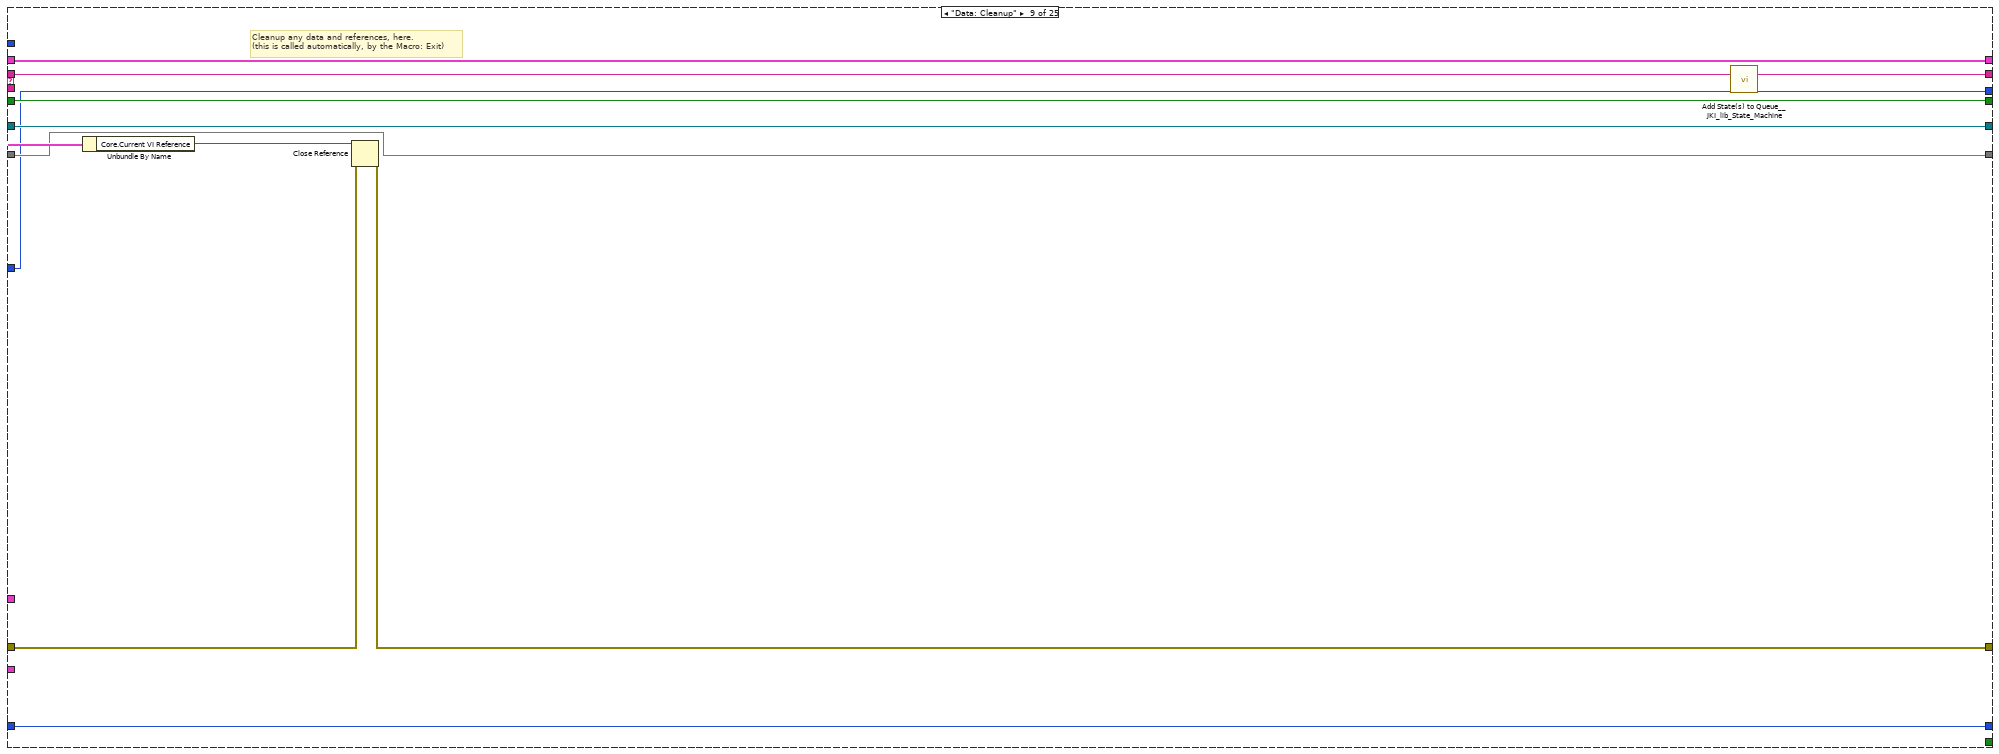
[diagram p17: hidden frame]
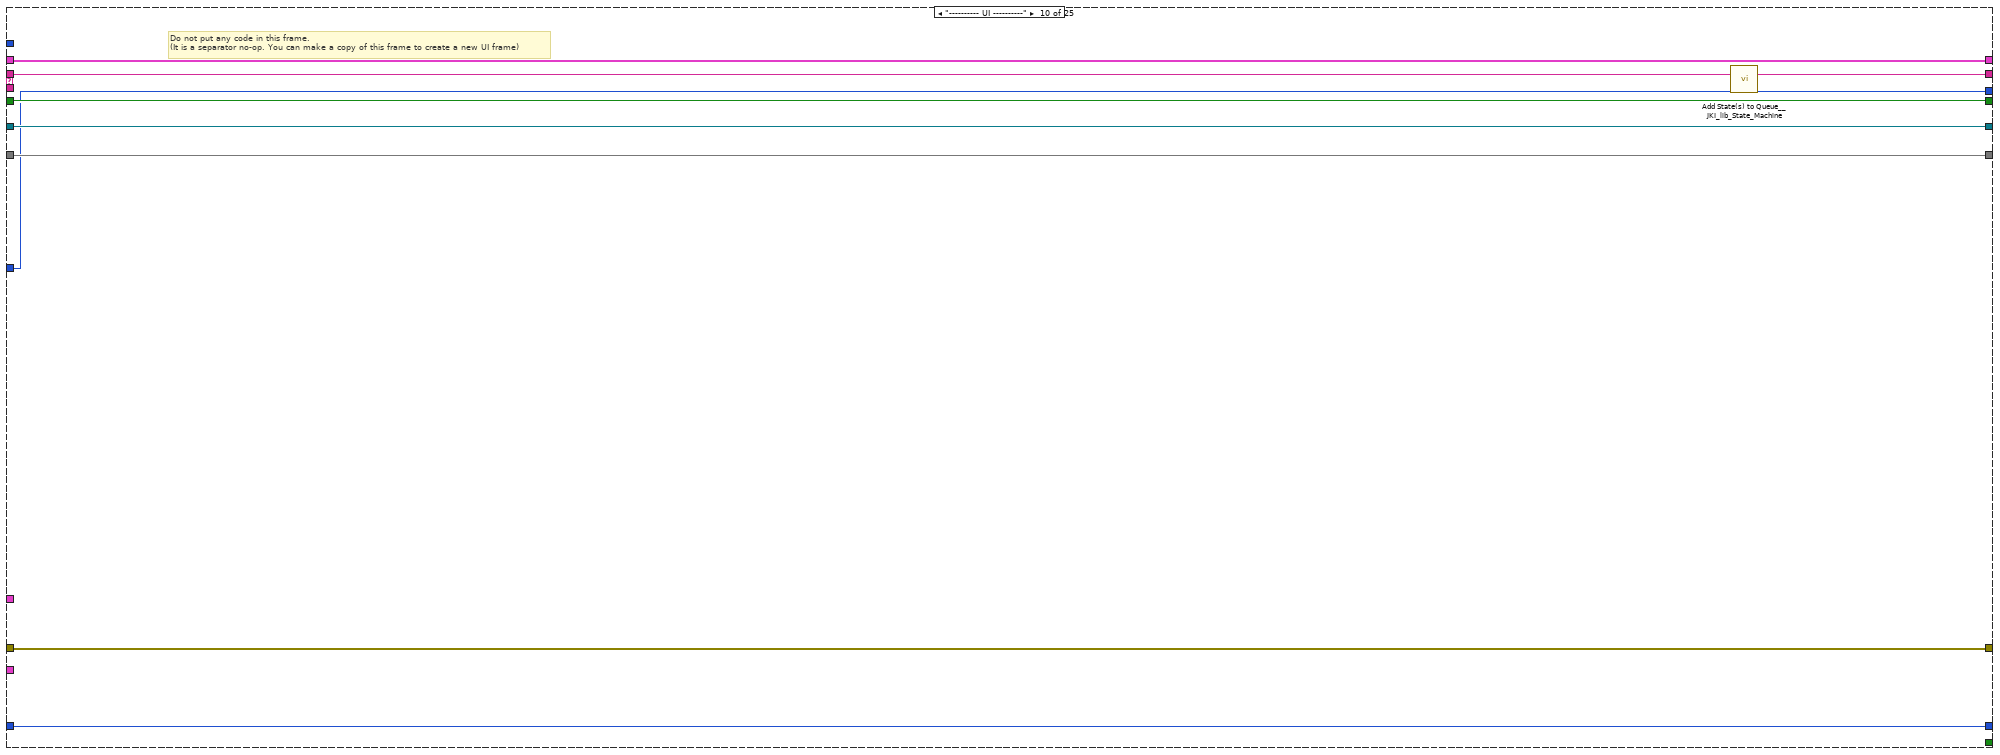
[diagram p18: hidden frame]
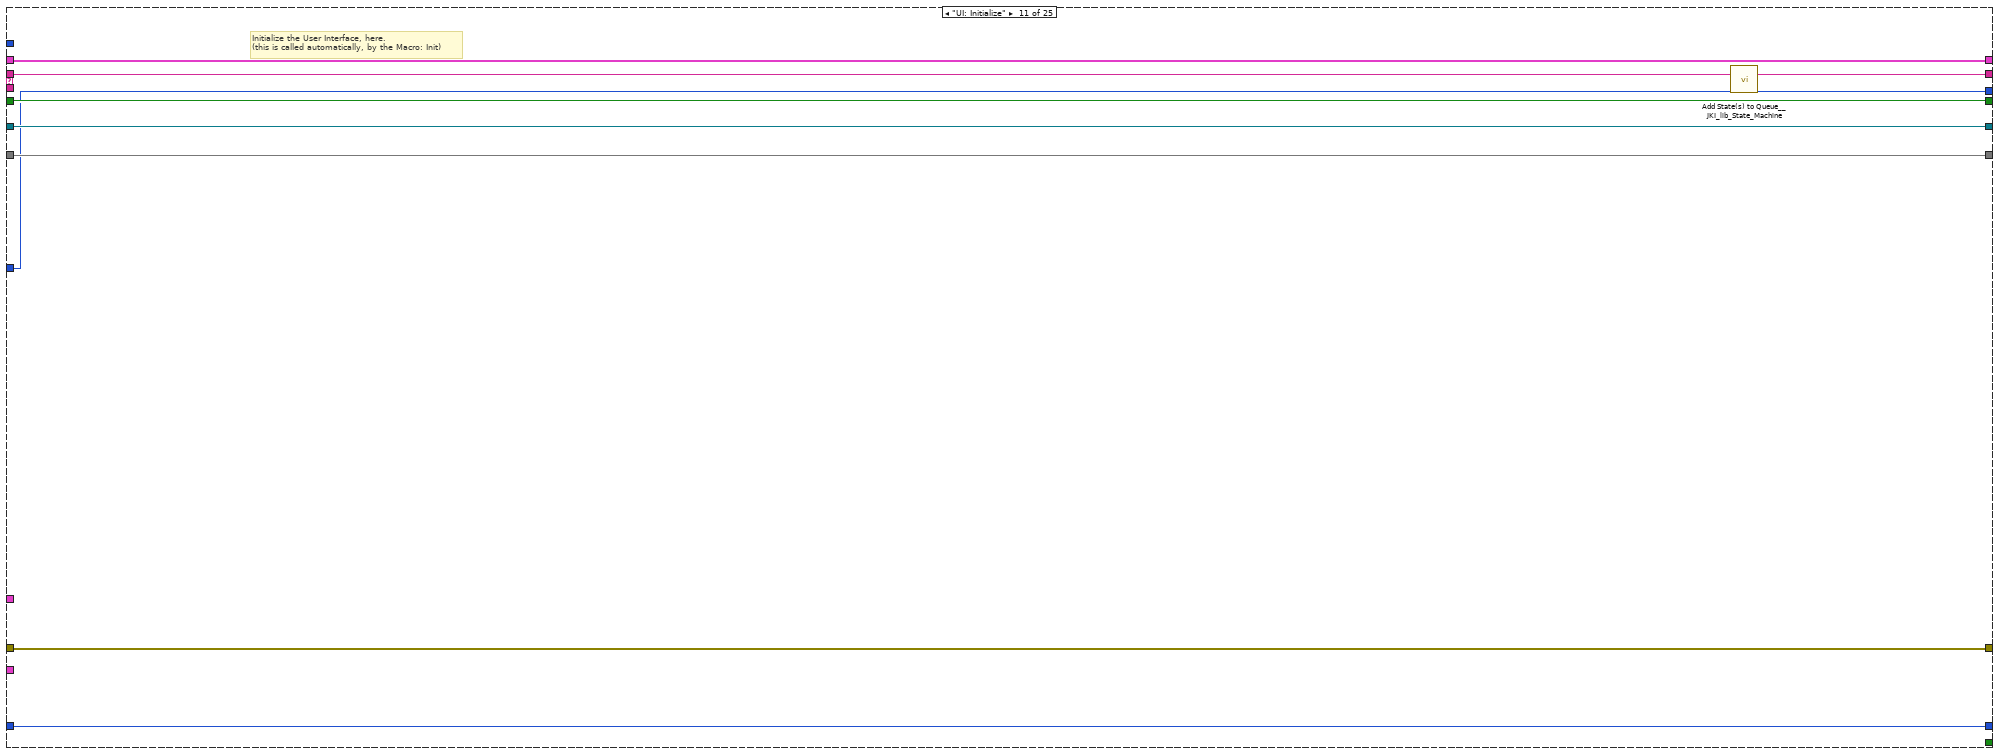
[diagram p19: hidden frame]
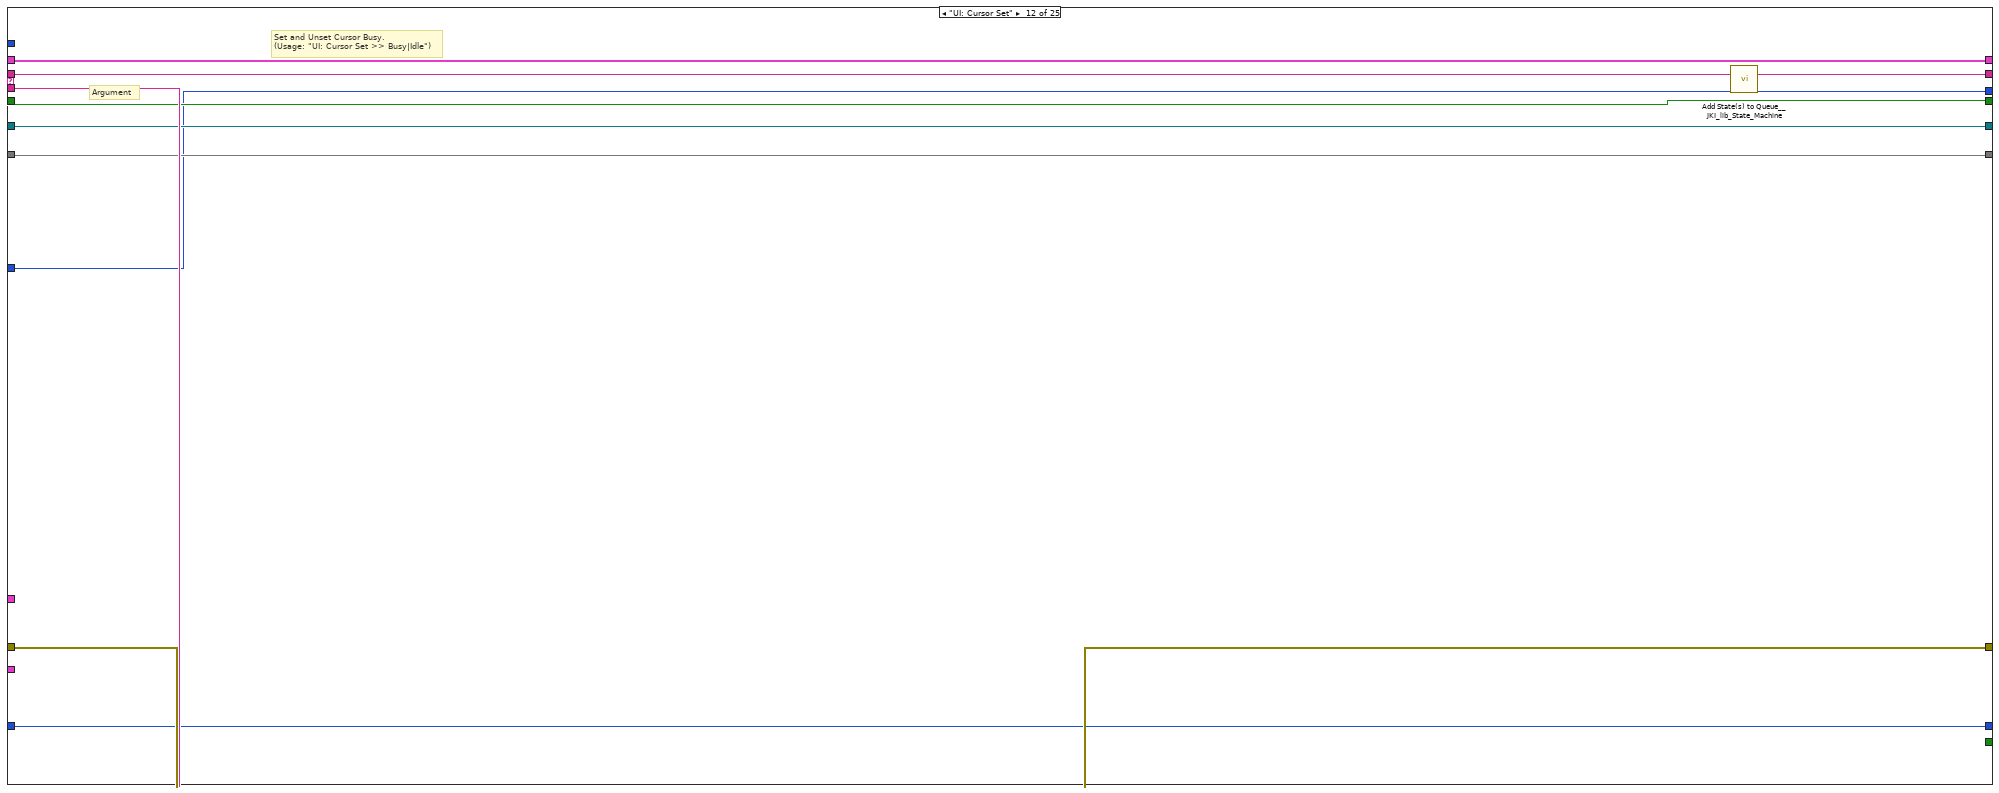
[diagram p20: hidden frame]
diagram:
  # "Register Required Events"
  # "Algo to dequeue the data from inspection ui and update the 2d array according to the JSON config data"
  n1 = Unbundle By Name("User Event References") -> ("Getdata"=w19:refnum<user-event>, "Analytics"=w18:refnum<user-event>, "Back"=w17:refnum<user-event>, "Stop_Analytics"=w16:refnum<user-event>, "Exit_Analytics"=w15:refnum<user-event>, "Pause_M"=w4:refnum<user-event>, "Override JSON"=w14:refnum<user-event>, "Initialization"=w13:refnum<user-event>)
  n2 = register-events(error in="error in", w19, w18, w17, w16, w15, w4, w14, w13) -> (reference out=w7:refnum<event-registration>, error out=w10:errorcluster)  [unwired: 1 in]
  n3 = call <vilib>:"Add State(s) to Queue__JKI_lib_State_Machine.vi"("State(s) in (\"\")"="Macro: Initialize") -> ("States Out"=w21:string)  [unwired: 14 in]
  n4 = while "JKI - String-Based Queued State Machine (Basic) v1.0" {
    shift-right: [w41] -> _
    shift-left: _ -> [w40]
    shift-right: [w44] -> w5
    shift-left: w10 -> [w36]
    shift-right: [w43] -> _
    shift-left: w21 -> [w45]
    tunnel: "Reference For PLot" -> [w38]
    shift-right: [w32] -> _
    shift-left: 0 -> [w37]
    tunnel: w7 -> [w34]
    tunnel: [w33] -> w6
    shift-right: [w31] -> _
    shift-left: FALSE -> [w35]
    shift-right: [w30] -> _
    shift-left: string[][] [["0"]] ("Statistical Parameters") -> [w29]
    shift-right: [w27] -> _
    shift-left: 0 -> [w28]
    tunnel: "Cluster Of Graphs" -> [w26]
    stop <- w42 stop-if-true
    w39 = -1  # Timeout
    n5 = call <vilib>:"Parse State Queue__JKI_lib_State_Machine.vi"("State Queue"=w45, "Error In (no error)"=w36) -> ("Remaining States"=w47:string, "Current State"=w48:string, "Arguments"=w46:string)  [unwired: 11 in]
    n6 = case shown="\"Analytics : GetData\"" w48 {
      selector: w48 -> [_ _ w163 _ _ _ _ _ _ _ _ _ _ _ _ _ _ _ _ _ _ _ _ _ _]
      tunnel: w47 -> [w56 w157 w167 w190 w201 w211 w220 w240 w251 w260 w269 w280 w296 w327 w337 w352 w361 w430 w514 w521 w554 w577 w589 w695 w706]
      tunnel: w46 -> [_ _ _ _ _ _ _ _ _ _ _ w275 w290 _ _ _ _ _ _ _ _ _ _ _ _]
      tunnel: w40 -> [w57 w154 w165 w181 w198 w209 w217 _ w246 w257 w267 w278 w292 w324 w334 w349 w358 w382 w507 w524 w549 w574 w591 w693 w704]
      tunnel: [w58 w155 w169 w187 errorcluster {"status"=FALSE, "code"=0, "source"=""} ("error out") w208 w218 w237 w247 w258 w266 w276 w293 w325 w335 w350 w359 w373 w512 w536 w540 w582 w600 w699 w709] -> w44
      tunnel: w36 -> [w59 w155 w168 w187 w197 w208 w218 w237 w248 w258 w266 w277 w294 w325 w335 w350 w359 w374 w512 w536 w546 w582 w600 w699 w709]
      tunnel: [w54 w156 w166 w189 w200 w210 w219 w239 w250 w259 w268 w279 w295 w326 w336 w351 w360 w429 w513 w520 w553 w576 w588 w694 w707] -> w43
      tunnel: [FALSE _ _ _ _ TRUE _ _ _ _ _ _ _ _ _ _ _ FALSE FALSE FALSE FALSE FALSE FALSE FALSE TRUE] -> w42
      tunnel: [w55 w154 w165 w188 w198 w209 w217 w238 w246 w257 w267 w278 w292 w324 w334 w349 w358 w394 w505 w522 w549 w578 w590 w692 w704] -> w41
      tunnel: w39 -> [_ _ _ _ _ _ _ _ _ _ _ _ _ _ _ _ _ _ _ _ _ _ _ _ _]
      tunnel: w38 -> [w63 _ _ _ _ _ _ _ _ _ _ _ _ _ _ _ _ w401 _ _ w548 _ _ _ _]
      tunnel: w37 -> [w52 w153 w162 w178 w195 w206 w216 w235 w245 w256 w265 w274 w289 w323 w332 w342 w357 w428 w503 w537 w556 w583 w631 w700 w710]
      tunnel: w35 -> [w62 w151 w160 w176 w193 w204 w214 w233 w243 w254 w263 w272 w287 w321 w330 w340 w355 w426 w510 w535 w555 w581 w630 w698 w708]
      tunnel: w34 -> [w61 w152 w161 w177 w194 w205 w215 w234 w244 w255 w264 w273 w288 w322 w331 w341 w356 w427 w511 w538 w557 w584 w632 w701 w711]
      tunnel: [w60 w152 w161 w177 w194 w205 w215 w234 w244 w255 w264 w273 w288 w322 w331 w341 w356 w427 w511 w538 w557 w584 w632 w701 w711] -> w33
      tunnel: [w52 w153 w162 w178 w195 w206 w216 w235 w245 w256 w265 w274 w289 w323 w332 w342 w357 w428 w502 w537 w556 w583 w631 w700 w710] -> w32
      tunnel: [w53 w151 w160 w176 w193 w204 w214 w233 w243 w254 w263 w272 w287 w321 w330 w340 w355 w426 w510 w535 w555 w581 w630 w698 w708] -> w31
      tunnel: [w51 w150 w159 w175 w192 w203 w213 w227 w242 w253 w262 w271 w286 w320 w329 w339 w354 w384 w493 w518 string[][] [] ("Statistical Parameters") w565 w586 w669 w703] -> w30
      tunnel: w29 -> [w51 w150 w159 w175 w192 w203 w213 w227 w242 w253 w262 w271 w286 w320 w329 w339 w354 w383 w493 w518 w545 w565 w586 w669 w703]
      tunnel: w28 -> [w49 w149 w158 w174 w191 w202 w212 w224 w241 w252 w261 w270 w285 w319 w328 w338 w353 w377 w492 w517 w539 w564 w585 w668 w702]
      tunnel: [w49 w149 w158 w174 w191 w202 w212 w224 w241 w252 w261 w270 w285 w319 w328 w338 w353 w376 w492 w517 w539 w564 w585 w668 w702] -> w27
      tunnel: w26 -> [_ _ _ _ _ _ _ _ _ _ _ _ _ _ _ _ _ w375 _ _ _ _ _ _ _]
      frame "", "Event Structure", "Idle" {
        n7 = event shown="[3] <Pause_M>: User Event" {
          selector: w61 -> [_ _ _ w96 w111 _ _ w143]
          dyn-events: [_ _ _ w95 w110 _ _ w142] -> w60
          timeout: _ -> [_ _ _ _ _ _ _ _]
          tunnel: [w64 w82 w88 w97 w112 w118 w129 w144] -> w58
          tunnel: w59 -> [w64 w82 w88 w98 w109 w118 w130 w148]
          tunnel: [TRUE TRUE FALSE FALSE FALSE FALSE w134 FALSE] -> w53
          tunnel: w62 -> [w75 _ _ _ _ _ w134 _]
          tunnel: w63 -> [_ _ _ _ w107 _ _ w141]
          tunnel: w57 -> [w66 w80 w86 w91 w103 w116 w124 w138]
          tunnel: w56 -> [w73 w78 w84 w93 w101 w120 w126 w136]
          tunnel: [w65 w80 w86 w90 w103 w114 w123 w138] -> w55
          tunnel: [w74 w77 w83 w92 w100 w119 w125 w135] -> w54
          event User Event {
            # "calculate execution time, Replace Array, Reduce Array"
            n8 = event-data() -> ("Terminal Count"=w71:u32, "isPass"=w70:bool, "Terminal Data 1D"=w69:dbl[], "Defect"=w68:bool[])  [unwired: 1 in]
            n9 = call <vilib>:"Add State(s) to Queue__JKI_lib_State_Machine.vi"("State(s) in Front (\"\")"="Analytics : GetData" ("State(s) in Front (\"\")"), "State(s) in (\"\")"=w73) -> ("States Out"=w74:string)  [unwired: 13 in]
            n10 = Bundle("Terminal Count"=w71, "isPass"=w70, "Terminal Data 1D"=w69, "Defect"=w68) -> (w67:T8)  [unwired: 1 in]
            n11 = Bundle By Name(cluster=w66, "REsultCluster"=w67) -> (w65:T11)
            "Get Data Active 2" <- w75
          }
          event User Event {
            # "Check if Analytics is pressed and set Boolean"
            n12 = event-data() -> ()  [unwired: 1 in, 1 out]
            n13 = call <vilib>:"Add State(s) to Queue__JKI_lib_State_Machine.vi"("State(s) in Front (\"\")"="Analytics : AnalyticsEvent" ("State(s) in Front (\"\")"), "State(s) in (\"\")"=w78) -> ("States Out"=w77:string)  [unwired: 13 in]
          }
          event User Event {
            # "Check if Back is pressed and reset Boolean"
            n14 = event-data() -> ()  [unwired: 1 in, 1 out]
            n15 = call <vilib>:"Add State(s) to Queue__JKI_lib_State_Machine.vi"("State(s) in Front (\"\")"="Analytics : Back" ("State(s) in Front (\"\")"), "State(s) in (\"\")"=w84) -> ("States Out"=w83:string)  [unwired: 13 in]
          }
          event User Event {
            # "Cp, CPk and Updated Graphs Displayed"
            n16 = event-data() -> ("Pause_M"=w89:bool)  [unwired: 1 in]
            n17 = Bundle By Name(cluster=w91, "Pause Data"=w89) -> (w90:T11)
            n18 = Flush Event Queue(0:w96, 3:w98) -> (8:w95:refnum<event-registration>, 11:w97:errorcluster)  [unwired: 4 in, 1 out]
            n19 = call <vilib>:"Add State(s) to Queue__JKI_lib_State_Machine.vi"("State(s) in Front (\"\")"="Analytics : PauseAnalytics" ("State(s) in Front (\"\")"), "State(s) in (\"\")"=w93) -> ("States Out"=w92:string)  [unwired: 13 in]
          }
          event User Event {
            # "Generate Stop For PLOT"
            # "Re-Initialize 2D Array to Zero values And flush event queue"
            n20 = event-data() -> ()  [unwired: 1 in, 1 out]
            n21 = Unbundle By Name(w107) -> ("Stop_Plot"=w106:refnum<user-event>)
            n22 = Generate User Event(priority (normal)=usereventprio."high priority", user event=w106, event data cluster=TRUE, error in=w109) -> (error out=w108:errorcluster)  [unwired: 1 out]
            n23 = Flush Event Queue(0:w111, 3:w108) -> (8:w110:refnum<event-registration>, 11:w112:errorcluster)  [unwired: 4 in, 1 out]
            n24 = call <vilib>:"Add State(s) to Queue__JKI_lib_State_Machine.vi"("State(s) in Front (\"\")"="Analytics : StopAnalytics" ("State(s) in Front (\"\")"), "State(s) in (\"\")"=w101) -> ("States Out"=w100:string)  [unwired: 13 in]
          }
          event User Event {
            # "Triggered with Pause  Button press"
            n25 = event-data() -> ("Initialization Values"=w115:T12)  [unwired: 1 in]
            n26 = call <vilib>:"Add State(s) to Queue__JKI_lib_State_Machine.vi"("State(s) in Front (\"\")"="Analytics : Initialization" ("State(s) in Front (\"\")"), "State(s) in (\"\")"=w120) -> ("States Out"=w119:string)  [unwired: 13 in]
            n27 = Bundle By Name(cluster=w116, "Initialization Values"=w115) -> (w114:T11)
          }
          event User Event {
            # "Triggerend with RUN button"
            n28 = event-data() -> ("JSON Path"=w131:path)  [unwired: 1 in]
            n29 = Read from Text File(file (use dialog)=w131, error in=w130) -> (text=w133:string, error out=w132:errorcluster)  [unwired: 2 in, 2 out]
            n30 = call "MainJSON.vi"("error in"=w132, "JSON String"=w133) -> ("error out"=w129:errorcluster, "Oveerride JSON DATATYPE"=w128:T13)  [unwired: 6 in, 2 out]
            n31 = Unbundle By Name(w128) -> ("AnalyticsDataFormat"=w122:T6)
            n32 = call <vilib>:"Add State(s) to Queue__JKI_lib_State_Machine.vi"("State(s) in Front (\"\")"="Analytics : OverrideJSON" ("State(s) in Front (\"\")"), "State(s) in (\"\")"=w126) -> ("States Out"=w125:string)  [unwired: 13 in]
            n33 = Bundle By Name(cluster=w124, "AnalyticsDataFormat"=w122) -> (w123:T11)
          }
          event User Event {
            # "Flush User Event Queue"
            # "Generate Exit User  Event for Plot Loop"
            n34 = event-data() -> ()  [unwired: 1 in, 1 out]
            n35 = Unbundle By Name(w141) -> ("Exit_PLot"=w140:refnum<user-event>)
            n36 = Generate User Event(priority (normal)=usereventprio."high priority", user event=w140, event data cluster=TRUE, error in=w148) -> (error out=w145:errorcluster)  [unwired: 1 out]
            n37 = Flush Event Queue(0:w143, 3:w145) -> (8:w142:refnum<event-registration>, 11:w144:errorcluster)  [unwired: 4 in, 1 out]
            n38 = call <vilib>:"Add State(s) to Queue__JKI_lib_State_Machine.vi"("State(s) in Front (\"\")"="Analytics : ExitAnalytics" ("State(s) in Front (\"\")"), "State(s) in (\"\")"=w136) -> ("States Out"=w135:string)  [unwired: 13 in]
          }
        }
      }
      frame "---------- Core ----------" {
        # "Do not put any code in this frame.\n(it is a separator no-op)"
        n39 = call <vilib>:"Add State(s) to Queue__JKI_lib_State_Machine.vi"("State(s) in (\"\")"=w157) -> ("States Out"=w156:string)  [unwired: 14 in]
      }
      frame Default {
        w172 = 42 items=["No error", "Argument error", "Memory is full", "Out of zone", "End of file", "File already open", "Generic file I/O error", "File not found", "File permission error", "Disk is full", "Duplicate path", "Too many files open", "System feature not enabled", "Resource file not found", "Cannot add resource", "Resource not found", "Image not found", "Image memory error", "Pen does not exist", "Config type invalid", "Config token not found", "Config parse error", "Config memory error", "Bad external code format", "Bad external code offset", "External code not present", "Null window", "Destroy window error", "Null menu", "Print aborted", "Bad print record", "Print driver error", "Windows error during printing", "Memory error during printing", "Print dialog error", "Generic print error", "Invalid device refnum", "Device not found", "Device parameter error", "Device unit error", "Cannot open device", "Device call aborted", "Generic error", "Cancelled by user", "Object ID too low", "Object ID too high", "Object not in heap", "Unknown heap", "Unknown object (invalid DefProc)", "Unknown object (DefProc not in table)", "Message out of range", "Invalid (null) method", "Unknown message", "Manager call not supported", "Bad address", "Network operation in progress", "Network operation timed out", "Connection is busy", "Network attribute not supported", "Network error", "Address in use", "System out of memory", "Connection aborted", "Connection refused", "Not connected", "Already connected", "Connection closed", "Initialization error (interapplication manager)", "Bad occurrence", "Wait on unbound occurrence handler", "Occurrence queue overflow", "Datalog type conflict", "Unused", "Unrecognized type (interapplication manager)", "Memory corrupt", "Failed to make temporary DLL", "Old CIN version", "Drag socket not found", "Failed to load drop-object", "Failed to register OLE object", "Failed to release OLE object", "Format specifier type mismatch", "Unknown format specifier", "Too few format specifiers", "Too many format specifiers", "Scan failed", "Newer CIN version", "Error converting to variant", "Runtime menu error", "Password tampered", "Variant attribute not found", "Incompatible variant data type", "Event data is not available", "Event Store is not present", "Occurrence is not found", "Event Queue is not created", "Event info is not available", "Refnum passed is NULL", "Error retrieving Class GUID", "Error retrieving CoClass GUID", "Error retrieving TypeLib GUID.", "Bad built application magic bytes.", "Specific driver is different from the specific driver associated with the Logical Name.", "There is no session opened to the class driver.", "Max Error", "MAX - Error with config objects", "MAX - Error loading configuration", "MAX - Group not supported"]
        # "Current State"
        # "Do not delete, rename, or modify this frame.\n(this is used to capture unhandled states and typos)"
        # "Handle mistyped state name (developer tool)"
        n40 = Format Into String(format string="Software Exception: Unhandled State \"%s\"." ("message"), error in=w168, w163) -> (resulting string=w171:string, error out=w170:errorcluster)  [unwired: 1 in]
        n41 = call <vilib>:"Error Cluster From Error Code.vi"("show call chain? (False)"=TRUE, "error in (no error)"=w170, "error message (\"\")"=w171, "error code (0)"=w172) -> ("error out"=w169:errorcluster)  [unwired: 5 in]
        n42 = call <vilib>:"Add State(s) to Queue__JKI_lib_State_Machine.vi"("State(s) in (\"\")"=w167) -> ("States Out"=w166:string)  [unwired: 14 in]
      }
      frame "Initialize Core Data" {
        # "Do not delete, rename, or modify this frame.\n(this is used to determine panel behavior on exit)"
        # "originally closed?"
        # "exe?"
        # "If panel starts closed or is an EXE, then close it when we exit"
        n43 = property class="VI"() -> ("Front Panel.Open"=w186:bool)  [unwired: 2 in, 2 out]
        n44 = property class="App"() -> ("App.Kind"=w185:T5)  [unwired: 2 in, 2 out]
        n45 = control-ref of="Current VI Reference"() -> (w179:refnum<vi>)
        n46 = Not(x=w186) -> (.not. x?=w183:bool)
        n47 = Equal?(x=w185, y=T5."Run Time System" ("Application:Kind")) -> (x = y?=w182:bool)
        n48 = Or(x=w183, y=w182) -> (x .or. y?=w180:bool)
        n49 = Bundle By Name(cluster=w181, "Core.Current VI Reference"=w179, "Core.Close Panel on Exit?"=w180) -> (w188:T11)
        n50 = call <vilib>:"Add State(s) to Queue__JKI_lib_State_Machine.vi"("State(s) in (\"\")"=w190) -> ("States Out"=w189:string)  [unwired: 14 in]
      }
      frame "Error Handler" {
        # "Unhandled Error -- Display it"
        # "Handle any errors here.\nYou can also output any states to clean-up after errors occur"
        # "Clear error"
        n51 = call <vilib>:"General Error Handler.vi"("error in (no error)"=w197) -> ()  [unwired: 10 in, 5 out]
        n52 = call <vilib>:"Add State(s) to Queue__JKI_lib_State_Machine.vi"("State(s) in Front (\"\")"="/* Post Error States", "State(s) in (\"\")"=w201) -> ("States Out"=w200:string)  [unwired: 13 in]
      }
      frame "Exit" {
        # "Do not put any code in this frame.\n(No errors that occur here will be handled.)"
        n53 = call <vilib>:"Add State(s) to Queue__JKI_lib_State_Machine.vi"("State(s) in (\"\")"=w211) -> ("States Out"=w210:string)  [unwired: 14 in]
      }
      frame "---------- Data ----------" {
        # "Do not put any code in this frame.\n(It is a separator no-op. You can make a copy of this frame to create a new Data frame)"
        n54 = call <vilib>:"Add State(s) to Queue__JKI_lib_State_Machine.vi"("State(s) in (\"\")"=w220) -> ("States Out"=w219:string)  [unwired: 14 in]
      }
      frame "Data: Initialize" {
        w221 = T14 {"InitializationDefect"=[0.0, 0.0, 0.0, 0.0, 0.0, 0.0, 0.0, 0.0, 0.0, 0.0, 0.0, 0.0, 0.0, 0.0, 0.0, 0.0, 0.0, 0.0, 0.0, 0.0, 0.0, 0.0, 0.0, 0.0, 0.0, 0.0, 0.0, 0.0, 0.0, 0.0, 0.0, 0.0, 0.0, 0.0, 0.0, 0.0, 0.0, 0.0, 0.0, 0.0, 0.0, 0.0, 0.0, 0.0, 0.0, 0.0, 0.0, 0.0, 0.0, 0.0, 0.0, 0.0, 0.0, 0.0, 0.0, 0.0, 0.0, 0.0, 0.0, 0.0, 0.0, 0.0, 0.0, 0.0, 0.0, 0.0, 0.0, 0.0, 0.0, 0.0, 0.0, 0.0, 0.0, 0.0, 0.0, 0.0, 0.0, 0.0, 0.0, 0.0, 0.0, 0.0, 0.0, 0.0, 0.0, 0.0, 0.0, 0.0, 0.0, 0.0, 0.0, 0.0, 0.0, 0.0, 0.0, 0.0, 0.0, 0.0, 0.0, 0.0, 0.0, 0.0, 0.0, 0.0, 0.0, 0.0, 0.0, 0.0, 0.0, 0.0, 0.0, 0.0, 0.0, 0.0, 0.0, 0.0, 0.0, 0.0, 0.0, 0.0, 0.0, 0.0, 0.0, 0.0, 0.0, 0.0, 0.0, 0.0, 0.0, 0.0, 0.0, 0.0, 0.0, 0.0, 0.0, 0.0, 0.0, 0.0, 0.0, 0.0, 0.0, 0.0, 0.0, 0.0, 0.0, 0.0, 0.0, 0.0, 0.0, 0.0, 0.0, 0.0, 0.0, 0.0, 0.0, 0.0, 0.0, 0.0, 0.0, 0.0, 0.0, 0.0, 0.0, 0.0, 0.0, 0.0, 0.0, 0.0, 0.0, 0.0, 0.0, 0.0, 0.0, 0.0, 0.0, 0.0, 0.0, 0.0, 0.0, 0.0, 0.0, 0.0, 0.0, 0.0, 0.0, 0.0, 0.0, 0.0, 0.0, 0.0, 0.0, 0.0, 0.0, 0.0, 0.0, 0.0, 0.0, 0.0, 0.0, 0.0, 0.0, 0.0, 0.0, 0.0, 0.0, 0.0, 0.0, 0.0, 0.0, 0.0, 0.0, 0.0, 0.0, 0.0, 0.0, 0.0, 0.0, 0.0, 0.0, 0.0, 0.0, 0.0, 0.0, 0.0, 0.0, 0.0, 0.0, 0.0, 0.0, 0.0, 0.0, 0.0, 0.0, 0.0, 0.0, 0.0, 0.0, 0.0, 0.0, 0.0, 0.0, 0.0, 0.0, 0.0, 0.0, 0.0, 0.0, 0.0, 0.0, 0.0, 0.0, 0.0, 0.0, 0.0, 0.0, 0.0, 0.0, 0.0, 0.0, 0.0, 0.0, 0.0, 0.0, 0.0, 0.0, 0.0, 0.0, 0.0, 0.0, 0.0, 0.0, 0.0, 0.0, 0.0, 0.0, 0.0, 0.0, 0.0, 0.0, 0.0, 0.0, 0.0, 0.0, 0.0, 0.0, 0.0, 0.0, 0.0, 0.0, 0.0, 0.0, 0.0, 0.0, 0.0, 0.0, 0.0, 0.0, 0.0, 0.0, 0.0, 0.0, 0.0, 0.0, 0.0, 0.0, 0.0, 0.0, 0.0, 0.0, 0.0, 0.0, 0.0, 0.0, 0.0, 0.0, 0.0, 0.0, 0.0, 0.0, 0.0, 0.0, 0.0, 0.0, 0.0, 0.0, 0.0, 0.0, 0.0, 0.0, 0.0, 0.0, 0.0, 0.0, 0.0, 0.0, 0.0, 0.0, 0.0, 0.0, 0.0, 0.0, 0.0, 0.0, 0.0, 0.0, 0.0, 0.0, 0.0, 0.0, 0.0, 0.0, 0.0, 0.0, 0.0, 0.0, 0.0, 0.0, 0.0, 0.0, 0.0, 0.0, 0.0, 0.0, 0.0, 0.0, 0.0, 0.0, 0.0, 0.0, 0.0, 0.0, 0.0, 0.0, 0.0, 0.0, 0.0, 0.0, 0.0, 0.0, 0.0, 0.0, 0.0, 0.0, 0.0, 0.0, 0.0, 0.0, 0.0, 0.0, 0.0, 0.0, 0.0, 0.0, 0.0, 0.0, 0.0, 0.0, 0.0, 0.0, 0.0, 0.0, 0.0, 0.0, 0.0, 0.0, 0.0, 0.0, 0.0, 0.0, 0.0, 0.0, 0.0, 0.0, 0.0, 0.0, 0.0, 0.0, 0.0, 0.0, 0.0, 0.0, 0.0, 0.0, 0.0, 0.0, 0.0, 0.0, 0.0, 0.0, 0.0, 0.0, 0.0, 0.0, 0.0, 0.0, 0.0, 0.0, 0.0, 0.0, 0.0, 0.0, 0.0, 0.0, 0.0, 0.0, 0.0, 0.0, 0.0, 0.0, 0.0, 0.0, 0.0, 0.0, 0.0, 0.0, 0.0, 0.0, 0.0, 0.0, 0.0, 0.0, 0.0, 0.0, 0.0, 0.0, 0.0, 0.0, 0.0, 0.0, 0.0, 0.0, 0.0, 0.0, 0.0, 0.0, 0.0, 0.0, 0.0, 0.0, 0.0, 0.0, 0.0, 0.0, 0.0, 0.0, 0.0, 0.0, 0.0, 0.0, 0.0, 0.0, 0.0, 0.0, 0.0, 0.0, 0.0, 0.0, 0.0, 0.0, 0.0, 0.0], "InitializationProduction"=[0.0, 0.0, 0.0, 0.0, 0.0, 0.0, 0.0, 0.0, 0.0, 0.0, 0.0, 0.0, 0.0, 0.0, 0.0, 0.0, 0.0, 0.0, 0.0, 0.0, 0.0]}  # InitializationValue-Barplot
        w222 = T14 {"InitializationDefect"=[0.0, 0.0, 0.0, 0.0, 0.0, 0.0, 0.0, 0.0, 0.0, 0.0, 0.0, 0.0, 0.0, 0.0, 0.0, 0.0, 0.0, 0.0, 0.0, 0.0, 0.0, 0.0, 0.0, 0.0, 0.0, 0.0, 0.0, 0.0, 0.0, 0.0, 0.0, 0.0, 0.0, 0.0, 0.0, 0.0, 0.0, 0.0, 0.0, 0.0, 0.0, 0.0, 0.0, 0.0, 0.0, 0.0, 0.0, 0.0, 0.0, 0.0, 0.0, 0.0, 0.0, 0.0, 0.0, 0.0, 0.0, 0.0, 0.0, 0.0, 0.0, 0.0, 0.0, 0.0, 0.0, 0.0, 0.0, 0.0, 0.0, 0.0, 0.0, 0.0, 0.0, 0.0, 0.0, 0.0, 0.0, 0.0, 0.0, 0.0, 0.0, 0.0, 0.0, 0.0, 0.0, 0.0, 0.0, 0.0, 0.0, 0.0, 0.0, 0.0, 0.0, 0.0, 0.0, 0.0, 0.0, 0.0, 0.0, 0.0, 0.0, 0.0, 0.0, 0.0, 0.0, 0.0, 0.0, 0.0, 0.0, 0.0, 0.0, 0.0, 0.0, 0.0, 0.0, 0.0, 0.0, 0.0, 0.0, 0.0, 0.0, 0.0, 0.0, 0.0, 0.0, 0.0, 0.0, 0.0, 0.0, 0.0, 0.0, 0.0, 0.0, 0.0, 0.0, 0.0, 0.0, 0.0, 0.0, 0.0, 0.0, 0.0, 0.0, 0.0, 0.0, 0.0, 0.0, 0.0, 0.0, 0.0, 0.0, 0.0, 0.0, 0.0, 0.0, 0.0, 0.0, 0.0, 0.0, 0.0, 0.0, 0.0, 0.0, 0.0, 0.0, 0.0, 0.0, 0.0, 0.0, 0.0, 0.0, 0.0, 0.0, 0.0, 0.0, 0.0, 0.0, 0.0, 0.0, 0.0, 0.0, 0.0, 0.0, 0.0, 0.0, 0.0, 0.0, 0.0, 0.0, 0.0, 0.0, 0.0, 0.0, 0.0, 0.0, 0.0, 0.0, 0.0, 0.0, 0.0, 0.0, 0.0, 0.0, 0.0, 0.0, 0.0, 0.0, 0.0, 0.0, 0.0, 0.0, 0.0, 0.0, 0.0, 0.0, 0.0, 0.0, 0.0, 0.0, 0.0, 0.0, 0.0, 0.0, 0.0, 0.0, 0.0, 0.0, 0.0, 0.0, 0.0, 0.0, 0.0, 0.0, 0.0, 0.0, 0.0, 0.0, 0.0, 0.0, 0.0, 0.0, 0.0, 0.0, 0.0, 0.0, 0.0, 0.0, 0.0, 0.0, 0.0, 0.0, 0.0, 0.0, 0.0, 0.0, 0.0, 0.0, 0.0, 0.0, 0.0, 0.0, 0.0, 0.0, 0.0, 0.0, 0.0, 0.0, 0.0, 0.0, 0.0, 0.0, 0.0, 0.0, 0.0, 0.0, 0.0, 0.0, 0.0, 0.0, 0.0, 0.0, 0.0, 0.0, 0.0, 0.0, 0.0, 0.0, 0.0, 0.0, 0.0, 0.0, 0.0, 0.0, 0.0, 0.0, 0.0, 0.0, 0.0, 0.0, 0.0, 0.0, 0.0, 0.0, 0.0, 0.0, 0.0, 0.0, 0.0, 0.0, 0.0, 0.0, 0.0, 0.0, 0.0, 0.0, 0.0, 0.0, 0.0, 0.0, 0.0, 0.0, 0.0, 0.0, 0.0, 0.0, 0.0, 0.0, 0.0, 0.0, 0.0, 0.0, 0.0, 0.0, 0.0, 0.0, 0.0, 0.0, 0.0, 0.0, 0.0, 0.0, 0.0, 0.0, 0.0, 0.0, 0.0, 0.0, 0.0, 0.0, 0.0, 0.0, 0.0, 0.0, 0.0, 0.0, 0.0, 0.0, 0.0, 0.0, 0.0, 0.0, 0.0, 0.0, 0.0, 0.0, 0.0, 0.0, 0.0, 0.0, 0.0, 0.0, 0.0, 0.0, 0.0, 0.0, 0.0, 0.0, 0.0, 0.0, 0.0, 0.0, 0.0, 0.0, 0.0, 0.0, 0.0, 0.0, 0.0, 0.0, 0.0, 0.0, 0.0, 0.0, 0.0, 0.0, 0.0, 0.0, 0.0, 0.0, 0.0, 0.0, 0.0, 0.0, 0.0, 0.0, 0.0, 0.0, 0.0, 0.0, 0.0, 0.0, 0.0, 0.0, 0.0, 0.0, 0.0, 0.0, 0.0, 0.0, 0.0, 0.0, 0.0, 0.0, 0.0, 0.0, 0.0, 0.0, 0.0, 0.0, 0.0, 0.0, 0.0, 0.0, 0.0, 0.0, 0.0, 0.0, 0.0, 0.0, 0.0, 0.0, 0.0, 0.0, 0.0, 0.0, 0.0, 0.0, 0.0, 0.0, 0.0, 0.0, 0.0, 0.0, 0.0, 0.0, 0.0, 0.0, 0.0, 0.0, 0.0, 0.0, 0.0, 0.0, 0.0, 0.0, 0.0, 0.0, 0.0, 0.0, 0.0, 0.0, 0.0, 0.0, 0.0, 0.0, 0.0, 0.0, 0.0, 0.0, 0.0, 0.0, 0.0, 0.0, 0.0, 0.0, 0.0, 0.0, 0.0, 0.0, 0.0, 0.0, 0.0, 0.0, 0.0, 0.0, 0.0, 0.0, 0.0, 0.0, 0.0, 0.0], "InitializationProduction"=[0.0, 0.0, 0.0, 0.0, 0.0, 0.0, 0.0, 0.0, 0.0, 0.0, 0.0, 0.0, 0.0, 0.0, 0.0, 0.0, 0.0, 0.0, 0.0, 0.0, 0.0]}  # InitializationValue-PieCahrt
        w223 = dbl[][] array501x21[10521 elements]  # InitializationValues
        w225 = string[][] [[" "]]  # Statistical Parameters
        w226 = TRUE  # Pause Data
        w229 = T8 {"Terminal Count"=0, "isPass"=FALSE, "Terminal Data 1D"=[], "Defect"=[]}  # REsultCluster
        w230 = T12 {"InitializationParams"={"CurrentPartNumber"="", "MeasurementData"=[]}}  # Initialization Values
        w231 = T10 {"Rows In 2D Array"=0, "Columns In 2D Array"=0, "Samples To Display"=0, "Update Rate (Time)"=0, "Update Rate (Samples)"=0, "MeasurementData"=[], "CurrentPartNumber"="", "AnalyticsDataFormat"={"AnalyticsParameters"={"UpdateRateCategories"={"LOW"={"SampleElapsed"=0, "TimeElapsed"=0}, "MEDIUM"={"SampleElapsed"=0, "TimeElapsed"=0}, "HIGH"={"SampleElapsed"=0, "TimeElapsed"=0}}, "AnalyticsForPartsList"=[]}}, "PlotParameters"={"Trend"=[], "Histogram"=[], "BarPlot"=[], "PieChart"=[]}}  # JSON Cluster
        w232 = T9 {"Initialize 2D Array"=[], "Analytics Button Pressed?"=FALSE, "Analytics Or Back?"=FALSE, "Read Config"=TRUE, "Prev Terminal Count"=0, "Plot:Present Terminal"=0, "Timeout?"=FALSE, "Re-initialized"=FALSE}  # clusterForShiftReg
        w236 = T15 {"Current VI Reference"=refnum, "Close Panel on Exit?"=FALSE}  # Core
        # "do not delete - used by framework"
        # "Data names and types of shift register data are defined by this bundle."
        # "Initialize the shift-register data, here.\n(data names are defined by what you wire into the bundle function)"
        n55 = Bundle("Core"=w236, "clusterForShiftReg"=w232, "JSON Cluster"=w231, "AnalyticsDataFormat"=T6 {"AnalyticsParameters"={"UpdateRateCategories"={"LOW"={"SampleElapsed"=0, "TimeElapsed"=0}, "MEDIUM"={"SampleElapsed"=0, "TimeElapsed"=0}, "HIGH"={"SampleElapsed"=0, "TimeElapsed"=0}}, "AnalyticsForPartsList"=[]}}, "Initialization Values"=w230, "REsultCluster"=w229, "Pause Data"=w226, "Statistical Parameters"=w225, "InitializationValues"=w223, "InitializationValue-PieCahrt"=w222, "InitializationValue-Barplot"=w221) -> (w238:T11)  [unwired: 1 in]
        n56 = call <vilib>:"Add State(s) to Queue__JKI_lib_State_Machine.vi"("State(s) in (\"\")"=w240) -> ("States Out"=w239:string)  [unwired: 14 in]
      }
      frame "Data: Cleanup" {
        # "Cleanup any data and references, here.\n(this is called automatically, by the Macro: Exit)"
        n57 = Unbundle By Name(w246) -> ("Core.Current VI Reference"=w249:refnum<vi>)
        n58 = Close Reference(reference=w249, error in (no error)=w248) -> (error out=w247:errorcluster)
        n59 = call <vilib>:"Add State(s) to Queue__JKI_lib_State_Machine.vi"("State(s) in (\"\")"=w251) -> ("States Out"=w250:string)  [unwired: 14 in]
      }
      frame "---------- UI ----------" {
        # "Do not put any code in this frame.\n(It is a separator no-op. You can make a copy of this frame to create a new UI frame)"
        n60 = call <vilib>:"Add State(s) to Queue__JKI_lib_State_Machine.vi"("State(s) in (\"\")"=w260) -> ("States Out"=w259:string)  [unwired: 14 in]
      }
      frame "UI: Initialize" {
        # "Initialize the User Interface, here.\n(this is called automatically, by the Macro: Init)"
        n61 = call <vilib>:"Add State(s) to Queue__JKI_lib_State_Machine.vi"("State(s) in (\"\")"=w269) -> ("States Out"=w268:string)  [unwired: 14 in]
      }
      frame "UI: Cursor Set" {
        # "Argument"
        # "Set and Unset Cursor Busy.\n(Usage: \"UI: Cursor Set >> Busy|Idle\")"
        n62 = case shown="\"Idle\", Default" w275 {
          tunnel: w277 -> [w282 w284]
          tunnel: [w281 w283] -> w276
          frame "Idle", Default {
            n63 = call <vilib>:"Unset Busy.vi"("error in (no error)"=w282) -> ("error out"=w281:errorcluster)  [unwired: 10 in]
          }
          frame "Busy" {
            n64 = call <vilib>:"Set Busy.vi"("error in (no error)"=w284) -> ("error out"=w283:errorcluster)  [unwired: 9 in, 1 out]
          }
        }
        n65 = call <vilib>:"Add State(s) to Queue__JKI_lib_State_Machine.vi"("State(s) in (\"\")"=w280) -> ("States Out"=w279:string)  [unwired: 14 in]
      }
      frame "UI: Front Panel State" {
        # "Argument"
        # "Set Front Panel Open or Closed\n(Usage: \"UI: Front Panel State >> Open|Close\")"
        n66 = Unbundle By Name(w292) -> ("Core.Current VI Reference"=w291:refnum<vi>)
        n67 = case shown="\"Close\"" w290 {
          tunnel: w294 -> [w300 w313]
          tunnel: [w302 w314] -> w293
          tunnel: w291 -> [w301 w311]
          frame "Open", Default {
            n68 = property class="VI"(reference=w301, error in=w300) -> (reference out=w298:refnum<vi>, error out=w299:errorcluster, "Front Panel.Open"=w297:bool)
            n69 = case shown="False" w297 {
              tunnel: [w305 w308] -> w302
              tunnel: w299 -> [w304 w308]
              tunnel: w298 -> [w303 _]
              frame False {
                n70 = invoke class="VI" method="FP.Open"(reference=w303, error in=w304, "Activate"=TRUE, "State"=T7."Standard") -> (error out=w305:errorcluster)  [unwired: 1 in, 4 out]
              }
              frame True {
              }
            }
          }
          frame "Close" {
            n71 = property class="VI"(reference=w311, error in=w313) -> (reference out=w310:refnum<vi>, error out=w312:errorcluster, "Front Panel.Open"=w309:bool)
            n72 = case shown="True" w309 {
              tunnel: [w315 w318] -> w314
              tunnel: w312 -> [w315 w317]
              tunnel: w310 -> [_ w316]
              frame False {
              }
              frame True {
                n73 = invoke class="VI" method="FP.Open"(reference=w316, error in=w317) -> (error out=w318:errorcluster)  [unwired: 3 in, 4 out]
              }
            }
          }
        }
        n74 = call <vilib>:"Add State(s) to Queue__JKI_lib_State_Machine.vi"("State(s) in (\"\")"=w296) -> ("States Out"=w295:string)  [unwired: 14 in]
      }
      frame "---------- Macro ----------" {
        # "Do not put any code in this frame.\n(It is a separator no-op. You can make a copy of this frame to create a new Macro frame)"
        n75 = call <vilib>:"Add State(s) to Queue__JKI_lib_State_Machine.vi"("State(s) in (\"\")"=w327) -> ("States Out"=w326:string)  [unwired: 14 in]
      }
      frame "Macro: Initialize" {
        w333 = "Data: Initialize\nInitialize Core Data\nUI: Initialize\nUI: Front Panel State >> Close"  # Data: Initialize Initialize Core Data UI: Initialize UI: Front Panel State >> Close
        # "Initialization Macro\n(This is called once, when the VI starts)"
        n76 = call <vilib>:"Add State(s) to Queue__JKI_lib_State_Machine.vi"("State(s) in Front (\"\")"=w333, "State(s) in (\"\")"=w337) -> ("States Out"=w336:string)  [unwired: 13 in]
      }
      frame "Macro: Exit" {
        # "Exit Macro\n(This is called once, when the VI exits)"
        n77 = Unbundle By Name(w349) -> ("Core.Close Panel on Exit?"=w348:bool)
        n78 = Select(t="UI: Front Panel State >> Close", s=w348, f="") -> (s? t:f=w345:string)
        n79 = call <vilib>:"Add State(s) to Queue__JKI_lib_State_Machine.vi"("State(s) in (\"\")"=w345, "State(s) at Back (\"\")"="Data: Cleanup\nExit") -> ("States Out"=w343:string)  [unwired: 13 in]
        n80 = call <vilib>:"Add State(s) to Queue__JKI_lib_State_Machine.vi"("State(s) in Front (\"\")"=w343, "State(s) in (\"\")"=w352) -> ("States Out"=w351:string)  [unwired: 13 in]
      }
      frame "---------- Analytics----------" {
        # "Template Separator\n(You can make a copy of, or modify, this frame)"
        n81 = call <vilib>:"Add State(s) to Queue__JKI_lib_State_Machine.vi"("State(s) in (\"\")"=w361) -> ("States Out"=w360:string)  [unwired: 14 in]
      }
      frame "Analytics : GetData" {
        w424 = T9 {"Initialize 2D Array"=[], "Analytics Button Pressed?"=FALSE, "Analytics Or Back?"=FALSE, "Read Config"=FALSE, "Prev Terminal Count"=0, "Plot:Present Terminal"=0, "Timeout?"=FALSE, "Re-initialized"=FALSE}  # Cluster For Shift Register
        # "calculate execution time, Replace Array, Reduce Array"
        # "Your code here.\n(You can make a copy of, or modify, this frame)"
        n82 = Unbundle By Name(w382) -> ("clusterForShiftReg"=w402:T9, "JSON Cluster"=w398:T10, "REsultCluster"=w397:T8, "InitializationValues"=w367:dbl[][], "InitializationValue-PieCahrt"=w366:T14, "InitializationValue-Barplot"=w365:T14)
        n83 = Unbundle By Name(w398) -> ("CurrentPartNumber"=w380:string, "Samples To Display"=w415:i32, "Rows In 2D Array"=w423:i32, "Update Rate (Time)"=w413:i32, "Update Rate (Samples)"=w412:i32, "PlotParameters"=w421:T16, "MeasurementData"=w392:T17)
        n84 = Unbundle By Name(w402) -> ("Initialize 2D Array"=w425:dbl[][], "Timeout?"=w409:bool, "Analytics Or Back?"=w411:bool, "Analytics Button Pressed?"=w410:bool, "Read Config"=w417:bool, "Re-initialized"=w403:bool, "Prev Terminal Count"=w404:u32, "Plot:Present Terminal"=w405:u32)
        n85 = Unbundle By Name(w397) -> ("Terminal Count"=w379:u32, "isPass"=w385:bool, "Terminal Data 1D"=w396:dbl[], "Defect"=w395:bool[])
        n86 = call "AnalyticsParamCluster.vi"("error in (no error)"=w374, "MeasurementData"=w392) -> ("error out"=w388:errorcluster, "Initialized Values"=w386:T18)  [unwired: 8 in]
        n87 = call "Concatenate to 1D.vi"("error in (no error)"=w374, "Defect"=w395, "Terminal Data 1D"=w396, "isPass"=w385) -> ("error out"=w420:errorcluster, "1D Concatenated Array"=w419:dbl[])  [unwired: 6 in]
        n88 = call "Replace and Reduce Array.vi"("dimension size"=w423, "initialized 2D in"=w425, "error in"=w420, "rows to display"=w415, "tc"=w379, "1D array"=w419) -> ("error out"=w390:errorcluster, "start index"=w416:i32, "reduced 2D"=w387:dbl[][], "initialized 2D out"=w418:dbl[][])  [unwired: 2 in]
        n89 = call "Cp-Cpk-SD-Mean-Variance-Calc.vi"("error in (no error)"=w390, "Initialized Values"=w386, "Reduced2DArray"=w387) -> ("error out"=w389:errorcluster, "Statistical Parameters"=w381:string[][])  [unwired: 7 in]
        n90 = Number To Decimal String(number=w379) -> (decimal integer string=w378:string)  [unwired: 1 in]
        n91 = Merge Errors(w389, w388) -> (w391:errorcluster)
        n92 = case shown="False" w385 {
          tunnel: w381 -> [w473 _]
          tunnel: [w471 string[][] [] ("Statistical Parameters")] -> w384
          tunnel: w383 -> [w486 _]
          tunnel: w380 -> [w484 _]
          tunnel: w378 -> [w483 _]
          tunnel: w377 -> [w470 w490]
          tunnel: [w469 w490] -> w376
          frame False {
            n93 = Get Date/Time In Seconds() -> (seconds since 1Jan1904=w482:timestamp)
            n94 = Index Array(array=w473, index (col)=0 ("disabled index (col)")) -> (element=w477:string[])  [unwired: 1 in]
            n95 = Get Date/Time String(seconds (now)=w482) -> (date string=w481:string, time string=w480:string)  [unwired: 2 in]
            n96 = Concatenate Strings(w481, " " ("string"), w480) -> (w478:string)
            n97 = Array Size(array=w477) -> (size(s)=w468:i32)
            n98 = for {
              N: w468 -> [_]
              tunnel: [w489] -> w475 mode=indexing
              tunnel: [w488] -> w474 mode=indexing
              tunnel: w484 -> [w489]
              tunnel: w483 -> [w488]
              tunnel: [w487] -> w472 mode=indexing
              tunnel: w478 -> [w487]
            }
            n99 = Insert Into Array(array=w486, index (row)=w470, new element #1=w475, new element #2=w474, new element #3=w473, new element #4=w472) -> (w485:string[][])  [unwired: 1 in]
            n100 = Transpose 2D Array(2D array=w485) -> (transposed array=w471:string[][])
            n101 = Add(x=w470, y=w468) -> (x+y=w469:i32)
          }
          frame True {
          }
        }
        n102 = call "Samples Elapsed.vi"("error in (no error)"=w391, "SE"=w412, "TC"=w379, "Plot:Present Terminal"=w404) -> ("error out"=w370:errorcluster, "Samples Elapsed"=w371:bool)  [unwired: 6 in]
        n103 = Compound Arithmetic op=OR(w410, w409, w371) -> (w372:bool)
        n104 = case shown="True" w372 {
          tunnel: [w436 w450] -> w369
          tunnel: w387 -> [_ w441]
          tunnel: w416 -> [_ w464]
          tunnel: w421 -> [_ w467]
          tunnel: w392 -> [_ w466]
          tunnel: w398 -> [w438 w465]
          tunnel: [w438 w465] -> w399
          tunnel: [w437 w460] -> w414
          tunnel: w415 -> [_ w462]
          tunnel: w379 -> [_ w461]
          tunnel: w404 -> [w437 w456]
          tunnel: w370 -> [w436 w457]
          tunnel: [w435 w456] -> w408
          tunnel: w405 -> [w435 _]
          tunnel: w410 -> [_ w455]
          tunnel: [FALSE w454] -> w368
          tunnel: w403 -> [_ w453]
          tunnel: w401 -> [_ _]
          tunnel: w381 -> [_ w452]
          tunnel: w386 -> [_ w451]
          tunnel: w375 -> [_ w448]
          tunnel: w367 -> [w433 w447]
          tunnel: w366 -> [w431 w446]
          tunnel: w365 -> [w432 w445]
          tunnel: [w433 w444] -> w364
          tunnel: [w432 w443] -> w363
          tunnel: [w431 w442] -> w362
          frame False {
          }
          frame True {
            w439 = T19 {"Reduced 2D"=[], "Start Index"=0, "MeasurementData"=[], "No Of New Termnals"=0, "Top/Bottom"=FALSE, "Values Inserted"=0, "PlotParameters"={"Trend"=[], "Histogram"=[], "BarPlot"=[], "PieChart"=[]}, "Re-Initialised"=FALSE, "Statistical params"=[], "MeasurementData_IndexValues"={"Measurement-ID"=[], "Measurement-Enable"=[], "LSL"=[], "USL"=[]}}  # Plot Cluster
            w454 = TRUE  # Reset
            n105 = call "New Terminals Updated.vi"("Prev Terminal Count"=w456, "error in (no error)"=w457, "Analytics Button Pressed?"=w455, "Samples to display"=w462, "Terminal Count"=w461) -> ("error out"=w449:errorcluster, "Top/Bottom"=w458:bool, "Values Inserted"=w459:i32, "No Of New Terminals"=w463:i32, "Prev Terminal Count"=w460:i32)  [unwired: 2 in]
            n106 = Bundle By Name(cluster=w439, "Re-Initialised"=w453, "Reduced 2D"=w441, "Start Index"=w464, "PlotParameters"=w467, "MeasurementData"=w466, "No Of New Termnals"=w463, "Values Inserted"=w459, "Top/Bottom"=w458, "Statistical params"=w452, "MeasurementData_IndexValues"=w451) -> (w440:T19)
            n107 = call "Plot.vi"("InitializationValue-Input-Barplot"=w445, "InitializationValue-Input-PieCahrt"=w446, "error Input"=w449, "Initialization input"=w447, "Graph Refference's"=w448, "Plot Cluster"=w440) -> ("error output"=w450:errorcluster, "InitializationOutput"=w444:dbl[][], "InitializationValue-output-Barplot"=w443:T14, "InitializationValue-output-PieCahrt"=w442:T14)  [unwired: 2 in]
          }
        }
        n108 = call "Time Elapsed.vi"("error in (no error)"=w369, "TE"=w413, "Reset"=w368) -> ("error out"=w373:errorcluster, "Timeout"=w407:bool)  [unwired: 7 in]
        n109 = Bundle By Name(cluster=w424, "Initialize 2D Array"=w418, "Timeout?"=w407, "Analytics Or Back?"=w411, "Analytics Button Pressed?"=FALSE, "Read Config"=w417, "Prev Terminal Count"=w414, "Plot:Present Terminal"=w408, "Re-initialized"=FALSE) -> (w400:T9)
        n110 = Bundle By Name(cluster=w382, "clusterForShiftReg"=w400, "JSON Cluster"=w399, "Statistical Parameters"=w381, "InitializationValues"=w364, "InitializationValue-PieCahrt"=w362, "InitializationValue-Barplot"=w363) -> (w394:T11)
        n111 = call <vilib>:"Add State(s) to Queue__JKI_lib_State_Machine.vi"("State(s) in (\"\")"=w430) -> ("States Out"=w429:string)  [unwired: 14 in]
      }
      frame "Analytics : AnalyticsEvent" {
        w501 = TRUE
        w508 = T9 {"Initialize 2D Array"=[], "Analytics Button Pressed?"=FALSE, "Analytics Or Back?"=FALSE, "Read Config"=FALSE, "Prev Terminal Count"=0, "Plot:Present Terminal"=0, "Timeout?"=FALSE, "Re-initialized"=FALSE}  # Cluster for Shift Register
        n112 = Unbundle By Name(w507) -> ("clusterForShiftReg"=w509:T9)
        n113 = Unbundle By Name(w509) -> ("Read Config"=w499:bool, "Initialize 2D Array"=w498:dbl[][], "Timeout?"=w497:bool, "Prev Terminal Count"=w496:u32, "Plot:Present Terminal"=w495:u32)
        n114 = Equal To 0?(x=w503) -> (x = 0?=w504:bool)
        n115 = Increment(x=w503) -> (x+1=w502:i32)
        n116 = case shown="True" w504 {
          tunnel: [FALSE TRUE] -> w500
          frame False {
          }
          frame True {
          }
        }
        n117 = Bundle By Name(cluster=w508, "Re-initialized"=w500, "Read Config"=w499, "Initialize 2D Array"=w498, "Timeout?"=w497, "Analytics Button Pressed?"=w501, "Analytics Or Back?"=w501, "Prev Terminal Count"=w496, "Plot:Present Terminal"=w495) -> (w506:T9)
        n118 = Bundle By Name(cluster=w507, "clusterForShiftReg"=w506) -> (w505:T11)
        n119 = call <vilib>:"Add State(s) to Queue__JKI_lib_State_Machine.vi"("State(s) in (\"\")"=w514) -> ("States Out"=w513:string)  [unwired: 14 in]
      }
      frame "Analytics : Back" {
        w525 = T9 {"Initialize 2D Array"=[], "Analytics Button Pressed?"=FALSE, "Analytics Or Back?"=FALSE, "Read Config"=FALSE, "Prev Terminal Count"=0, "Plot:Present Terminal"=0, "Timeout?"=FALSE, "Re-initialized"=FALSE}  # Cluster for Shift Register
        n120 = Unbundle By Name(w524) -> ("clusterForShiftReg"=w534:T9)
        n121 = Unbundle By Name(w534) -> ("Re-initialized"=w533:bool, "Initialize 2D Array"=w532:dbl[][], "Timeout?"=w531:bool, "Analytics Button Pressed?"=w530:bool, "Read Config"=w529:bool, "Prev Terminal Count"=w528:u32, "Plot:Present Terminal"=w527:u32)
        n122 = Bundle By Name(cluster=w525, "Re-initialized"=w533, "Initialize 2D Array"=w532, "Timeout?"=w531, "Analytics Button Pressed?"=w530, "Analytics Or Back?"=FALSE, "Read Config"=w529, "Prev Terminal Count"=w528, "Plot:Present Terminal"=w527) -> (w523:T9)
        n123 = Bundle By Name(cluster=w524, "clusterForShiftReg"=w523) -> (w522:T11)
        n124 = call <vilib>:"Add State(s) to Queue__JKI_lib_State_Machine.vi"("State(s) in (\"\")"=w521) -> ("States Out"=w520:string)  [unwired: 14 in]
      }
      frame "Analytics : PauseAnalytics" {
        n125 = Unbundle By Name(w549) -> ("Pause Data"=w550:bool, "Statistical Parameters"=w547:string[][])
        n126 = case shown="True" w550 {
          tunnel: w546 -> [w558 w561]
          tunnel: [w558 w560] -> w541
          tunnel: w548 -> [_ w563]
          tunnel: w547 -> [_ w559]
          frame False {
          }
          frame True {
            n127 = Unbundle By Name(w563) -> ("CpCpkData"=w562:refnum<user-event>)
            n128 = Generate User Event(user event=w562, event data cluster=w559, error in=w561) -> (error out=w560:errorcluster)  [unwired: 1 in, 1 out]
          }
        }
        n129 = call-poly <vilib>:"Write Delimited Spreadsheet.vi"("file path (dialog if empty)"=path "C:/Users/akshatav/Desktop/AnalyticsStatisticalData.csv", "2D data"=w545, "append to file? (F)"=TRUE ("append to file? (new file:F)"), "error in (no error)"=w541, "delimiter (\\t)"="," ("delimiter (\\t)")) -> ("error out"=w540:errorcluster)  [unwired: 9 in, 1 out]
        n130 = call <vilib>:"Add State(s) to Queue__JKI_lib_State_Machine.vi"("State(s) in (\"\")"=w554) -> ("States Out"=w553:string)  [unwired: 14 in]
      }
      frame "Analytics : StopAnalytics" {
        w568 = u32 0 ("Prev Terminal Count")
        w580 = T9 {"Initialize 2D Array"=[], "Analytics Button Pressed?"=FALSE, "Analytics Or Back?"=FALSE, "Read Config"=FALSE, "Prev Terminal Count"=0, "Plot:Present Terminal"=0, "Timeout?"=FALSE, "Re-initialized"=FALSE}  # Cluster for Shift Register
        n131 = Unbundle By Name(w574) -> ("clusterForShiftReg"=w575:T9)
        n132 = Unbundle By Name(w575) -> ("Re-initialized"=w573:bool, "Initialize 2D Array"=w572:dbl[][], "Timeout?"=w571:bool, "Analytics Button Pressed?"=w570:bool, "Analytics Or Back?"=w569:bool)
        n133 = Bundle By Name(cluster=w580, "Re-initialized"=w573, "Initialize 2D Array"=w572, "Timeout?"=w571, "Analytics Button Pressed?"=w570, "Analytics Or Back?"=w569, "Read Config"=TRUE, "Prev Terminal Count"=w568, "Plot:Present Terminal"=w568) -> (w579:T9)
        n134 = Bundle By Name(cluster=w574, "clusterForShiftReg"=w579) -> (w578:T11)
        n135 = call <vilib>:"Add State(s) to Queue__JKI_lib_State_Machine.vi"("State(s) in (\"\")"=w577) -> ("States Out"=w576:string)  [unwired: 14 in]
      }
      frame "Analytics : Initialization" {
        w596 = T10 {"Rows In 2D Array"=0, "Columns In 2D Array"=0, "Samples To Display"=0, "Update Rate (Time)"=0, "Update Rate (Samples)"=0, "MeasurementData"=[], "CurrentPartNumber"="", "AnalyticsDataFormat"={"AnalyticsParameters"={"UpdateRateCategories"={"LOW"={"SampleElapsed"=0, "TimeElapsed"=0}, "MEDIUM"={"SampleElapsed"=0, "TimeElapsed"=0}, "HIGH"={"SampleElapsed"=0, "TimeElapsed"=0}}, "AnalyticsForPartsList"=[]}}, "PlotParameters"={"Trend"=[], "Histogram"=[], "BarPlot"=[], "PieChart"=[]}}  # JSON Cluster
        w601 = T9 {"Initialize 2D Array"=[], "Analytics Button Pressed?"=FALSE, "Analytics Or Back?"=FALSE, "Read Config"=FALSE, "Prev Terminal Count"=0, "Plot:Present Terminal"=0, "Timeout?"=FALSE, "Re-initialized"=FALSE}  # Cluster For Shift Register
        # "Triggered with Pause  Button press"
        n136 = Unbundle By Name(w591) -> ("clusterForShiftReg"=w599:T9, "JSON Cluster"=w598:T10, "Initialization Values"=w594:T12, "JSON Cluster"=w592:T10)
        n137 = Unbundle By Name(w594) -> ("InitializationParams"=w593:T20)
        n138 = Unbundle By Name(w599) -> ("Re-initialized"=w629:bool, "Plot:Present Terminal"=w628:u32, "Prev Terminal Count"=w627:u32, "Initialize 2D Array"=w621:dbl[][], "Timeout?"=w602:bool, "Analytics Button Pressed?"=w603:bool, "Analytics Or Back?"=w604:bool, "Read Config"=w620:bool)
        n139 = Unbundle By Name(w593) -> ("MeasurementData"=w618:T17, "CurrentPartNumber"=w617:string)
        n140 = Unbundle By Name(w598) -> ("Rows In 2D Array"=w606:i32, "Samples To Display"=w607:i32, "Columns In 2D Array"=w608:i32, "Update Rate (Samples)"=w609:i32, "Update Rate (Time)"=w610:i32, "PlotParameters"=w605:T16, "CurrentPartNumber"=w623:string)
        n141 = case shown="True" w620 {
          tunnel: [w636 w653] -> _
          tunnel: w600 -> [w637 w660]
          tunnel: [w649 w667] -> w624
          tunnel: w618 -> [w649 w667]
          tunnel: [w643 w664] -> w615
          tunnel: [w642 w651] -> w616
          tunnel: [w641 w650] -> w612
          tunnel: [w633 w652] -> w611
          tunnel: w605 -> [_ _]
          tunnel: w606 -> [_ _]
          tunnel: w607 -> [_ _]
          tunnel: w608 -> [_ _]
          tunnel: w609 -> [_ _]
          tunnel: w610 -> [_ _]
          tunnel: [w640 w658] -> w613
          tunnel: [w639 w657] -> w614
          tunnel: w617 -> [_ w662]
          tunnel: [w648 w663] -> w622
          tunnel: w621 -> [w648 _]
          tunnel: w623 -> [w638 _]
          tunnel: [w638 w662] -> w625
          tunnel: [w635 w656] -> w626
          tunnel: w592 -> [w634 w655]
          frame False {
            n142 = call "Json_Specific part.vi"("error in (no error)"=w637, "JSON Cluster"=w634, "Part-num"=w638) -> ("error out"=w646:errorcluster, "Json Part no specicific op"=w647:T21)  [unwired: 7 in]
            n143 = Unbundle By Name(w647) -> ("Array Params.RowsIn2DArray"=w643:i32, "Array Params.SamplesToDisplay"=w642:i32, "Array Params.ColumnsIn2DArray"=w641:i32, "Array Params.UpdateRate"=w645:string, "PlotParameters"=w633:T16)
            n144 = call "String To Enum.vi"("error in (no error)"=w646, "string"=w645) -> ("error out"=w644:errorcluster, "Select Update Rate"=w635:enum16{"HIGH", "MEDIUM", "LOW"})  [unwired: 8 in]
            n145 = call "Rate to Sampls&Time.vi"("error in (no error)"=w644, "JSON Cluster"=w634, "Select Update Rate"=w635) -> ("error out"=w636:errorcluster, "TimeElapsed"=w639:i32, "SampleElapsed"=w640:i32)  [unwired: 6 in]
          }
          frame True {
            # "Triggered with Stop Button Press"
            n146 = call "Json_Specific part.vi"("error in (no error)"=w660, "JSON Cluster"=w655, "Part-num"=w662) -> ("error out"=w659:errorcluster, "Json Part no specicific op"=w661:T21)  [unwired: 7 in]
            n147 = Unbundle By Name(w661) -> ("Array Params.RowsIn2DArray"=w664:i32, "Array Params.SamplesToDisplay"=w651:i32, "Array Params.ColumnsIn2DArray"=w650:i32, "Array Params.UpdateRate"=w666:string, "PlotParameters"=w652:T16)
            n148 = call "String To Enum.vi"("error in (no error)"=w659, "string"=w666) -> ("error out"=w654:errorcluster, "Select Update Rate"=w656:enum16{"HIGH", "MEDIUM", "LOW"})  [unwired: 8 in]
            n149 = call "Rate to Sampls&Time.vi"("error in (no error)"=w654, "JSON Cluster"=w655, "Select Update Rate"=w656) -> ("error out"=w653:errorcluster, "TimeElapsed"=w657:i32, "SampleElapsed"=w658:i32)  [unwired: 6 in]
            n150 = Initialize Array(nan ("element"), w664, w650) -> (w663:dbl[][])
          }
        }
        "Default Update Rate  3" <- w626
        n151 = Bundle By Name(cluster=w601, "Re-initialized"=w629, "Plot:Present Terminal"=w628, "Prev Terminal Count"=w627, "Initialize 2D Array"=w622, "Timeout?"=w602, "Analytics Button Pressed?"=w603, "Analytics Or Back?"=w604, "Read Config"=FALSE) -> (w597:T9)
        n152 = Bundle By Name(cluster=w596, "Rows In 2D Array"=w615, "Samples To Display"=w616, "Columns In 2D Array"=w612, "Update Rate (Samples)"=w613, "Update Rate (Time)"=w614, "PlotParameters"=w611, "CurrentPartNumber"=w625, "MeasurementData"=w624) -> (w595:T10)
        n153 = call <vilib>:"Add State(s) to Queue__JKI_lib_State_Machine.vi"("State(s) in (\"\")"=w589) -> ("States Out"=w588:string)  [unwired: 14 in]
        n154 = Bundle By Name(cluster=w591, "clusterForShiftReg"=w597, "JSON Cluster"=w595) -> (w590:T11)
      }
      frame "Analytics : OverrideJSON" {
        w681 = T10 {"Rows In 2D Array"=0, "Columns In 2D Array"=0, "Samples To Display"=0, "Update Rate (Time)"=0, "Update Rate (Samples)"=0, "MeasurementData"=[], "CurrentPartNumber"="", "AnalyticsDataFormat"={"AnalyticsParameters"={"UpdateRateCategories"={"LOW"={"SampleElapsed"=0, "TimeElapsed"=0}, "MEDIUM"={"SampleElapsed"=0, "TimeElapsed"=0}, "HIGH"={"SampleElapsed"=0, "TimeElapsed"=0}}, "AnalyticsForPartsList"=[]}}, "PlotParameters"={"Trend"=[], "Histogram"=[], "BarPlot"=[], "PieChart"=[]}}  # JSON Cluster
        w696 = T9 {"Initialize 2D Array"=[], "Analytics Button Pressed?"=FALSE, "Analytics Or Back?"=FALSE, "Read Config"=FALSE, "Prev Terminal Count"=0, "Plot:Present Terminal"=0, "Timeout?"=FALSE, "Re-initialized"=FALSE}  # Cluster for Shift Register
        n155 = Unbundle By Name(w693) -> ("clusterForShiftReg"=w697:T9, "JSON Cluster"=w682:T10, "AnalyticsDataFormat"=w672:T6)
        n156 = Unbundle By Name(w697) -> ("Initialize 2D Array"=w689:dbl[][], "Timeout?"=w688:bool, "Analytics Button Pressed?"=w687:bool, "Analytics Or Back?"=w686:bool, "Read Config"=w685:bool, "Prev Terminal Count"=w684:u32, "Plot:Present Terminal"=w683:u32)
        n157 = Unbundle By Name(w682) -> ("Rows In 2D Array"=w680:i32, "Columns In 2D Array"=w679:i32, "Samples To Display"=w678:i32, "Update Rate (Time)"=w677:i32, "Update Rate (Samples)"=w676:i32, "PlotParameters"=w675:T16, "MeasurementData"=w674:T17, "CurrentPartNumber"=w673:string)
        n158 = Bundle By Name(cluster=w696, "Re-initialized"=TRUE, "Initialize 2D Array"=w689, "Timeout?"=w688, "Analytics Button Pressed?"=w687, "Analytics Or Back?"=w686, "Read Config"=w685, "Prev Terminal Count"=w684, "Plot:Present Terminal"=w683) -> (w691:T9)
        n159 = Bundle By Name(cluster=w681, "Rows In 2D Array"=w680, "Columns In 2D Array"=w679, "Samples To Display"=w678, "Update Rate (Time)"=w677, "Update Rate (Samples)"=w676, "PlotParameters"=w675, "MeasurementData"=w674, "CurrentPartNumber"=w673, "AnalyticsDataFormat"=w672) -> (w671:T10)
        n160 = call <vilib>:"Add State(s) to Queue__JKI_lib_State_Machine.vi"("State(s) in (\"\")"=w695) -> ("States Out"=w694:string)  [unwired: 14 in]
        n161 = Bundle By Name(cluster=w693, "clusterForShiftReg"=w691, "JSON Cluster"=w671) -> (w692:T11)
      }
      frame "Analytics : ExitAnalytics" {
        n162 = call <vilib>:"Add State(s) to Queue__JKI_lib_State_Machine.vi"("State(s) in (\"\")"=w706) -> ("States Out"=w707:string)  [unwired: 14 in]
      }
    }
  }
  n163 = Unregister For Events(event registration refnum=w6, error in=w5) -> (error out=w23:errorcluster)
  n164 = call "ErrorHandling.vi"("error in (no error)"=w23, "Vi-name"="GetData loop.vi") -> ("error out"=→"error out":errorcluster)  [unwired: 9 in]
